vi "test_Checksum U16 - Add Protection.vi"(8 "error in (no error)":errorcluster) -> (0 "error out":errorcluster)   [LabVIEW 2019, in "Protections Unit Tests.lvclass"]
uses:
  Protections Unit Tests.lvclass
  Checksum U16/Checksum U16.lvclass
  <vilib>/addons/_JKI Toolkits/VI Tester/TestCase.llb/TestCase.lvclass
  C:/Program Files (x86)/National Instruments/LabVIEW 2019/vi.lib/addons/_JKI Toolkits/VI Tester/TestCase.llb/TestCase.lvclass
panel:
  out "Checksum U16 out":refnum<class "Checksum U16.lvclass">
  in  "Checksum U16 in":refnum<class "Checksum U16.lvclass">
  out "TestCase out":refnum<class "Protections Unit Tests.lvclass">
  in  "TestCase in":refnum<class "Protections Unit Tests.lvclass">
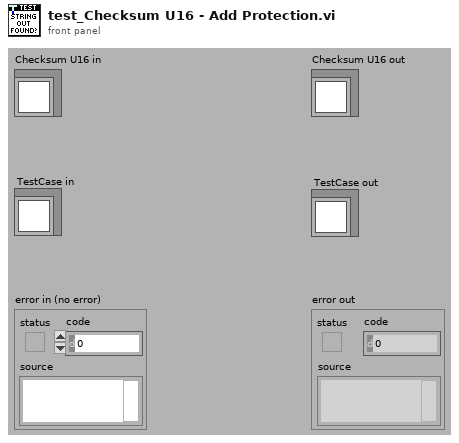
[diagram p1: front panel]
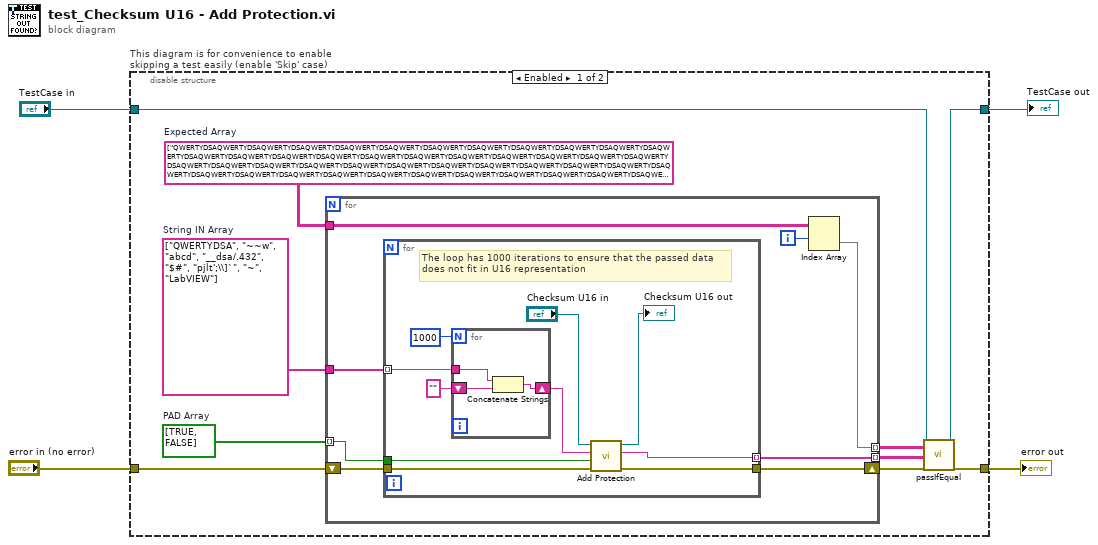
[diagram p0: block diagram]
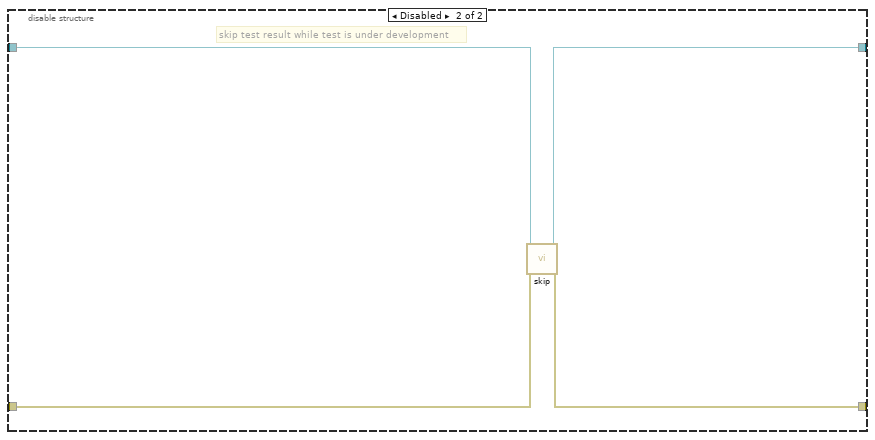
[diagram p2: hidden frame]
diagram:
  n1 = disable-structure "This diagram is for convenience to enable skipping a test easily (enable 'Skip' case)" shown="Enabled" {
    disable-tunnel: "TestCase in" -> [w12 w39]
    disable-tunnel: [w13 w37] -> w1
    disable-tunnel: [w14 w38] -> w3
    disable-tunnel: "error in (no error)" -> [w11 w36]
    frame Enabled {
      w6 = string[][] [["QWERTYDSAQWERTYDSAQWERTYDSAQWERTYDSAQWERTYDSAQWERTYDSAQWERTYDSAQWERTYDSAQWERTYDSAQWERTYDSAQWERTYDSAQWERTYDSAQWERTYDSAQWERTYDSAQWERTYDSAQWERTYDSAQWERTYDSAQWERTYDSAQWERTYDSAQWERTYDSAQWERTYDSAQWERTYDSAQWERTYDSAQWERTYDSAQWERTYDSAQWERTYDSAQWERTYDSAQWERTYDSAQWERTYDSAQWERTYDSAQWERTYDSAQWERTYDSAQWERTYDSAQWERTYDSAQWERTYDSAQWERTYDSAQWERTYDSAQWERTYDSAQWERTYDSAQWERTYDSAQWERTYDSAQWERTYDSAQWERTYDSAQWERTYDSAQWERTYDSAQWERTYDSAQWERTYDSAQWERTYDSAQWERTYDSAQWERTYDSAQWERTYDSAQWERTYDSAQWERTYDSAQWERTYDSAQWERTYDSAQWERTYDSAQWERTYDSAQWERTYDSAQWERTYDSAQWERTYDSAQWERTYDSAQWERTYDSAQWERTYDSAQWERTYDSAQWERTYDSAQWERTYDSAQWERTYDSAQWERTYDSAQWERTYDSAQWERTYDSAQWERTYDSAQWERTYDSAQWERTYDSAQWERTYDSAQWERTYDSAQWERTYDSAQWERTYDSAQWERTYDSAQWERTYDSAQWERTYDSAQWERTYDSAQWERTYDSAQWERTYDSAQWERTYDSAQWERTYDSAQWERTYDSAQWERTYDSAQWERTYDSAQWERTYDSAQWERTYDSAQWERTYDSAQWERTYDSAQWERTYDSAQWERTYDSAQWERTYDSAQWERTYDSAQWERTYDSAQWERTYDSAQWERTYDSAQWERTYDSAQWERTYDSAQWERTYDSAQWERTYDSAQWERTYDSAQWERTYDSAQWERTYDSAQWERTYDSAQWERTYDSAQWERTYDSAQWERTYDSAQWERTYDSAQWERTYDSAQWERTYDSAQWERTYDSAQWERTYDSAQWERTYDSAQWERTYDSAQWERTYDSAQWERTYDSAQWERTYDSAQWERTYDSAQWERTYDSAQWERTYDSAQWERTYDSAQWERTYDSAQWERTYDSAQWERTYDSAQWERTYDSAQWERTYDSAQWERTYDSAQWERTYDSAQWERTYDSAQWERTYDSAQWERTYDSAQWERTYDSAQWERTYDSAQWERTYDSAQWERTYDSAQWERTYDSAQWERTYDSAQWERTYDSAQWERTYDSAQWERTYDSAQWERTYDSAQWERTYDSAQWERTYDSAQWERTYDSAQWERTYDSAQWERTYDSAQWERTYDSAQWERTYDSAQWERTYDSAQWERTYDSAQWERTYDSAQWERTYDSAQWERTYDSAQWERTYDSAQWERTYDSAQWERTYDSAQWERTYDSAQWERTYDSAQWERTYDSAQWERTYDSAQWERTYDSAQWERTYDSAQWERTYDSAQWERTYDSAQWERTYDSAQWERTYDSAQWERTYDSAQWERTYDSAQWERTYDSAQWERTYDSAQWERTYDSAQWERTYDSAQWERTYDSAQWERTYDSAQWERTYDSAQWERTYDSAQWERTYDSAQWERTYDSAQWERTYDSAQWERTYDSAQWERTYDSAQWERTYDSAQWERTYDSAQWERTYDSAQWERTYDSAQWERTYDSAQWERTYDSAQWERTYDSAQWERTYDSAQWERTYDSAQWERTYDSAQWERTYDSAQWERTYDSAQWERTYDSAQWERTYDSAQWERTYDSAQWERTYDSAQWERTYDSAQWERTYDSAQWERTYDSAQWERTYDSAQWERTYDSAQWERTYDSAQWERTYDSAQWERTYDSAQWERTYDSAQWERTYDSAQWERTYDSAQWERTYDSAQWERTYDSAQWERTYDSAQWERTYDSAQWERTYDSAQWERTYDSAQWERTYDSAQWERTYDSAQWERTYDSAQWERTYDSAQWERTYDSAQWERTYDSAQWERTYDSAQWERTYDSAQWERTYDSAQWERTYDSAQWERTYDSAQWERTYDSAQWERTYDSAQWERTYDSAQWERTYDSAQWERTYDSAQWERTYDSAQWERTYDSAQWERTYDSAQWERTYDSAQWERTYDSAQWERTYDSAQWERTYDSAQWERTYDSAQWERTYDSAQWERTYDSAQWERTYDSAQWERTYDSAQWERTYDSAQWERTYDSAQWERTYDSAQWERTYDSAQWERTYDSAQWERTYDSAQWERTYDSAQWERTYDSAQWERTYDSAQWERTYDSAQWERTYDSAQWERTYDSAQWERTYDSAQWERTYDSAQWERTYDSAQWERTYDSAQWERTYDSAQWERTYDSAQWERTYDSAQWERTYDSAQWERTYDSAQWERTYDSAQWERTYDSAQWERTYDSAQWERTYDSAQWERTYDSAQWERTYDSAQWERTYDSAQWERTYDSAQWERTYDSAQWERTYDSAQWERTYDSAQWERTYDSAQWERTYDSAQWERTYDSAQWERTYDSAQWERTYDSAQWERTYDSAQWERTYDSAQWERTYDSAQWERTYDSAQWERTYDSAQWERTYDSAQWERTYDSAQWERTYDSAQWERTYDSAQWERTYDSAQWERTYDSAQWERTYDSAQWERTYDSAQWERTYDSAQWERTYDSAQWERTYDSAQWERTYDSAQWERTYDSAQWERTYDSAQWERTYDSAQWERTYDSAQWERTYDSAQWERTYDSAQWERTYDSAQWERTYDSAQWERTYDSAQWERTYDSAQWERTYDSAQWERTYDSAQWERTYDSAQWERTYDSAQWERTYDSAQWERTYDSAQWERTYDSAQWERTYDSAQWERTYDSAQWERTYDSAQWERTYDSAQWERTYDSAQWERTYDSAQWERTYDSAQWERTYDSAQWERTYDSAQWERTYDSAQWERTYDSAQWERTYDSAQWERTYDSAQWERTYDSAQWERTYDSAQWERTYDSAQWERTYDSAQWERTYDSAQWERTYDSAQWERTYDSAQWERTYDSAQWERTYDSAQWERTYDSAQWERTYDSAQWERTYDSAQWERTYDSAQWERTYDSAQWERTYDSAQWERTYDSAQWERTYDSAQWERTYDSAQWERTYDSAQWERTYDSAQWERTYDSAQWERTYDSAQWERTYDSAQWERTYDSAQWERTYDSAQWERTYDSAQWERTYDSAQWERTYDSAQWERTYDSAQWERTYDSAQWERTYDSAQWERTYDSAQWERTYDSAQWERTYDSAQWERTYDSAQWERTYDSAQWERTYDSAQWERTYDSAQWERTYDSAQWERTYDSAQWERTYDSAQWERTYDSAQWERTYDSAQWERTYDSAQWERTYDSAQWERTYDSAQWERTYDSAQWERTYDSAQWERTYDSAQWERTYDSAQWERTYDSAQWERTYDSAQWERTYDSAQWERTYDSAQWERTYDSAQWERTYDSAQWERTYDSAQWERTYDSAQWERTYDSAQWERTYDSAQWERTYDSAQWERTYDSAQWERTYDSAQWERTYDSAQWERTYDSAQWERTYDSAQWERTYDSAQWERTYDSAQWERTYDSAQWERTYDSAQWERTYDSAQWERTYDSAQWERTYDSAQWERTYDSAQWERTYDSAQWERTYDSAQWERTYDSAQWERTYDSAQWERTYDSAQWERTYDSAQWERTYDSAQWERTYDSAQWERTYDSAQWERTYDSAQWERTYDSAQWERTYDSAQWERTYDSAQWERTYDSAQWERTYDSAQWERTYDSAQWERTYDSAQWERTYDSAQWERTYDSAQWERTYDSAQWERTYDSAQWERTYDSAQWERTYDSAQWERTYDSAQWERTYDSAQWERTYDSAQWERTYDSAQWERTYDSAQWERTYDSAQWERTYDSAQWERTYDSAQWERTYDSAQWERTYDSAQWERTYDSAQWERTYDSAQWERTYDSAQWERTYDSAQWERTYDSAQWERTYDSAQWERTYDSAQWERTYDSAQWERTYDSAQWERTYDSAQWERTYDSAQWERTYDSAQWERTYDSAQWERTYDSAQWERTYDSAQWERTYDSAQWERTYDSAQWERTYDSAQWERTYDSAQWERTYDSAQWERTYDSAQWERTYDSAQWERTYDSAQWERTYDSAQWERTYDSAQWERTYDSAQWERTYDSAQWERTYDSAQWERTYDSAQWERTYDSAQWERTYDSAQWERTYDSAQWERTYDSAQWERTYDSAQWERTYDSAQWERTYDSAQWERTYDSAQWERTYDSAQWERTYDSAQWERTYDSAQWERTYDSAQWERTYDSAQWERTYDSAQWERTYDSAQWERTYDSAQWERTYDSAQWERTYDSAQWERTYDSAQWERTYDSAQWERTYDSAQWERTYDSAQWERTYDSAQWERTYDSAQWERTYDSAQWERTYDSAQWERTYDSAQWERTYDSAQWERTYDSAQWERTYDSAQWERTYDSAQWERTYDSAQWERTYDSAQWERTYDSAQWERTYDSAQWERTYDSAQWERTYDSAQWERTYDSAQWERTYDSAQWERTYDSAQWERTYDSAQWERTYDSAQWERTYDSAQWERTYDSAQWERTYDSAQWERTYDSAQWERTYDSAQWERTYDSAQWERTYDSAQWERTYDSAQWERTYDSAQWERTYDSAQWERTYDSAQWERTYDSAQWERTYDSAQWERTYDSAQWERTYDSAQWERTYDSAQWERTYDSAQWERTYDSAQWERTYDSAQWERTYDSAQWERTYDSAQWERTYDSAQWERTYDSAQWERTYDSAQWERTYDSAQWERTYDSAQWERTYDSAQWERTYDSAQWERTYDSAQWERTYDSAQWERTYDSAQWERTYDSAQWERTYDSAQWERTYDSAQWERTYDSAQWERTYDSAQWERTYDSAQWERTYDSAQWERTYDSAQWERTYDSAQWERTYDSAQWERTYDSAQWERTYDSAQWERTYDSAQWERTYDSAQWERTYDSAQWERTYDSAQWERTYDSAQWERTYDSAQWERTYDSAQWERTYDSAQWERTYDSAQWERTYDSAQWERTYDSAQWERTYDSAQWERTYDSAQWERTYDSAQWERTYDSAQWERTYDSAQWERTYDSAQWERTYDSAQWERTYDSAQWERTYDSAQWERTYDSAQWERTYDSAQWERTYDSAQWERTYDSAQWERTYDSAQWERTYDSAQWERTYDSAQWERTYDSAQWERTYDSAQWERTYDSAQWERTYDSAQWERTYDSAQWERTYDSAQWERTYDSAQWERTYDSAQWERTYDSAQWERTYDSAQWERTYDSAQWERTYDSAQWERTYDSAQWERTYDSAQWERTYDSAQWERTYDSAQWERTYDSAQWERTYDSAQWERTYDSAQWERTYDSAQWERTYDSAQWERTYDSAQWERTYDSAQWERTYDSAQWERTYDSAQWERTYDSAQWERTYDSAQWERTYDSAQWERTYDSAQWERTYDSAQWERTYDSAQWERTYDSAQWERTYDSAQWERTYDSAQWERTYDSAQWERTYDSAQWERTYDSAQWERTYDSAQWERTYDSAQWERTYDSAQWERTYDSAQWERTYDSAQWERTYDSAQWERTYDSAQWERTYDSAQWERTYDSAQWERTYDSAQWERTYDSAQWERTYDSAQWERTYDSAQWERTYDSAQWERTYDSAQWERTYDSAQWERTYDSAQWERTYDSAQWERTYDSAQWERTYDSAQWERTYDSAQWERTYDSAQWERTYDSAQWERTYDSAQWERTYDSAQWERTYDSAQWERTYDSAQWERTYDSAQWERTYDSAQWERTYDSAQWERTYDSAQWERTYDSAQWERTYDSAQWERTYDSAQWERTYDSAQWERTYDSAQWERTYDSAQWERTYDSAQWERTYDSAQWERTYDSAQWERTYDSAQWERTYDSAQWERTYDSAQWERTYDSAQWERTYDSAQWERTYDSAQWERTYDSAQWERTYDSAQWERTYDSAQWERTYDSAQWERTYDSAQWERTYDSAQWERTYDSAQWERTYDSAQWERTYDSAQWERTYDSAQWERTYDSAQWERTYDSAQWERTYDSAQWERTYDSAQWERTYDSAQWERTYDSAQWERTYDSAQWERTYDSAQWERTYDSAQWERTYDSAQWERTYDSAQWERTYDSAQWERTYDSAQWERTYDSAQWERTYDSAQWERTYDSAQWERTYDSAQWERTYDSAQWERTYDSAQWERTYDSAQWERTYDSAQWERTYDSAQWERTYDSAQWERTYDSAQWERTYDSAQWERTYDSAQWERTYDSAQWERTYDSAQWERTYDSAQWERTYDSAQWERTYDSAQWERTYDSAQWERTYDSAQWERTYDSAQWERTYDSAQWERTYDSAQWERTYDSAQWERTYDSAQWERTYDSAQWERTYDSAQWERTYDSAQWERTYDSAQWERTYDSAQWERTYDSAQWERTYDSAQWERTYDSAQWERTYDSAQWERTYDSAQWERTYDSAQWERTYDSAQWERTYDSAQWERTYDSAQWERTYDSAQWERTYDSAQWERTYDSAQWERTYDSAQWERTYDSAQWERTYDSAQWERTYDSAQWERTYDSAQWERTYDSAQWERTYDSAQWERTYDSAQWERTYDSAQWERTYDSAQWERTYDSAQWERTYDSAQWERTYDSAQWERTYDSAQWERTYDSAQWERTYDSAQWERTYDSAQWERTYDSAQWERTYDSAQWERTYDSAQWERTYDSAQWERTYDSAQWERTYDSAQWERTYDSAQWERTYDSAQWERTYDSAQWERTYDSAQWERTYDSAQWERTYDSAQWERTYDSAQWERTYDSAQWERTYDSAQWERTYDSAQWERTYDSAQWERTYDSAQWERTYDSAQWERTYDSAQWERTYDSAQWERTYDSAQWERTYDSAQWERTYDSAQWERTYDSAQWERTYDSAQWERTYDSAQWERTYDSAQWERTYDSAQWERTYDSAQWERTYDSAQWERTYDSAQWERTYDSAQWERTYDSAQWERTYDSAQWERTYDSAQWERTYDSAQWERTYDSAQWERTYDSAQWERTYDSAQWERTYDSAQWERTYDSAQWERTYDSAQWERTYDSAQWERTYDSAQWERTYDSAQWERTYDSAQWERTYDSAQWERTYDSAQWERTYDSAQWERTYDSAQWERTYDSAQWERTYDSAQWERTYDSAQWERTYDSAQWERTYDSAQWERTYDSAQWERTYDSAQWERTYDSAQWERTYDSAQWERTYDSAQWERTYDSAQWERTYDSAQWERTYDSAQWERTYDSAQWERTYDSAQWERTYDSAQWERTYDSAQWERTYDSAQWERTYDSAQWERTYDSAQWERTYDSAQWERTYDSAQWERTYDSAQWERTYDSAQWERTYDSAQWERTYDSAQWERTYDSAQWERTYDSAQWERTYDSAQWERTYDSAQWERTYDSAQWERTYDSAQWERTYDSAQWERTYDSAQWERTYDSAQWERTYDSAQWERTYDSAQWERTYDSAQWERTYDSAQWERTYDSAQWERTYDSAQWERTYDSAQWERTYDSAQWERTYDSAQWERTYDSAQWERTYDSAQWERTYDSAQWERTYDSAQWERTYDSAQWERTYDSAQWERTYDSAQWERTYDSAQWERTYDSAQWERTYDSAQWERTYDSAQWERTYDSAQWERTYDSAQWERTYDSAQWERTYDSAQWERTYDSAQWERTYDSAQWERTYDSAQWERTYDSAQWERTYDSAQWERTYDSAQWERTYDSAQWERTYDSAQWERTYDSAQWERTYDSAQWERTYDSAQWERTYDSAQWERTYDSAQWERTYDSAQWERTYDSAQWERTYDSAQWERTYDSAQWERTYDSAQWERTYDSAQWERTYDSAQWERTYDSAQWERTYDSAQWERTYDSAQWERTYDSAQWERTYDSAQWERTYDSAQWERTYDSAQWERTYDSAQWERTYDSAQWERTYDSAQWERTYDSAQWERTYDSAQWERTYDSAQWERTYDSAQWERTYDSAQWERTYDSAQWERTYDSAQWERTYDSAQWERTYDSAQWERTYDSAQWERTYDSAQWERTYDSAQWERTYDSAQWERTYDSAQWERTYDSAQWERTYDSAQWERTYDSAQWERTYDSAQWERTYDSAQWERTYDSAQWERTYDSAQWERTYDSAQWERTYDSAQWERTYDSAQWERTYDSAQWERTYDSAQWERTYDSAQWERTYDSAQWERTYDSAQWERTYDSAQWERTYDSAQWERTYDSAQWERTYDSAQWERTYDSAQWERTYDSAQWERTYDSAQWERTYDSAQWERTYDSAQWERTYDSAQWERTYDSAQWERTYDSAQWERTYDSAQWERTYDSAQWERTYDSAQWERTYDSAQWERTYDSAQWERTYDSAQWERTYDSAQWERTYDSAQWERTYDSAQWERTYDSAQWERTYDSAQWERTYDSAQWERTYDSAQWERTYDSAQWERTYDSAQWERTYDSAQWERTYDSAQWERTYDSAQWERTYDSAQWERTYDSAQWERTYDSAQWERTYDSAQWERTYDSAQWERTYDSAQWERTYDSAQWERTYDSAQWERTYDSAQWERTYDSAQWERTYDSAQWERTYDSAQWERTYDSAQWERTYDSAQWERTYDSAQWERTYDSAQWERTYDSAQWERTYDSAQWERTYDSAQWERTYDSAQWERTYDSAQWERTYDSAQWERTYDSAQWERTYDSAQWERTYDSAQWERTYDSAQWERTYDSAQWERTYDSAQWERTYDSAQWERTYDSAQWERTYDSAQWERTYDSAQWERTYDSAQWERTYDSAQWERTYDSAQWERTYDSAQWERTYDSAQWERTYDSAQWERTYDSAQWERTYDSAQWERTYDSAQWERTYDSAQWERTYDSAQWERTYDSAQWERTYDSAQWERTYDSAQWERTYDSAQWERTYDSAQWERTYDSAQWERTYDSAQWERTYDSAQWERTYDSAQWERTYDSAQWERTYDSAQWERTYDSAQWERTYDSAQWERTYDSAQWERTYDSAQWERTYD͠", "~~w~~w~~w~~w~~w~~w~~w~~w~~w~~w~~w~~w~~w~~w~~w~~w~~w~~w~~w~~w~~w~~w~~w~~w~~w~~w~~w~~w~~w~~w~~w~~w~~w~~w~~w~~w~~w~~w~~w~~w~~w~~w~~w~~w~~w~~w~~w~~w~~w~~w~~w~~w~~w~~w~~w~~w~~w~~w~~w~~w~~w~~w~~w~~w~~w~~w~~w~~w~~w~~w~~w~~w~~w~~w~~w~~w~~w~~w~~w~~w~~w~~w~~w~~w~~w~~w~~w~~w~~w~~w~~w~~w~~w~~w~~w~~w~~w~~w~~w~~w~~w~~w~~w~~w~~w~~w~~w~~w~~w~~w~~w~~w~~w~~w~~w~~w~~w~~w~~w~~w~~w~~w~~w~~w~~w~~w~~w~~w~~w~~w~~w~~w~~w~~w~~w~~w~~w~~w~~w~~w~~w~~w~~w~~w~~w~~w~~w~~w~~w~~w~~w~~w~~w~~w~~w~~w~~w~~w~~w~~w~~w~~w~~w~~w~~w~~w~~w~~w~~w~~w~~w~~w~~w~~w~~w~~w~~w~~w~~w~~w~~w~~w~~w~~w~~w~~w~~w~~w~~w~~w~~w~~w~~w~~w~~w~~w~~w~~w~~w~~w~~w~~w~~w~~w~~w~~w~~w~~w~~w~~w~~w~~w~~w~~w~~w~~w~~w~~w~~w~~w~~w~~w~~w~~w~~w~~w~~w~~w~~w~~w~~w~~w~~w~~w~~w~~w~~w~~w~~w~~w~~w~~w~~w~~w~~w~~w~~w~~w~~w~~w~~w~~w~~w~~w~~w~~w~~w~~w~~w~~w~~w~~w~~w~~w~~w~~w~~w~~w~~w~~w~~w~~w~~w~~w~~w~~w~~w~~w~~w~~w~~w~~w~~w~~w~~w~~w~~w~~w~~w~~w~~w~~w~~w~~w~~w~~w~~w~~w~~w~~w~~w~~w~~w~~w~~w~~w~~w~~w~~w~~w~~w~~w~~w~~w~~w~~w~~w~~w~~w~~w~~w~~w~~w~~w~~w~~w~~w~~w~~w~~w~~w~~w~~w~~w~~w~~w~~w~~w~~w~~w~~w~~w~~w~~w~~w~~w~~w~~w~~w~~w~~w~~w~~w~~w~~w~~w~~w~~w~~w~~w~~w~~w~~w~~w~~w~~w~~w~~w~~w~~w~~w~~w~~w~~w~~w~~w~~w~~w~~w~~w~~w~~w~~w~~w~~w~~w~~w~~w~~w~~w~~w~~w~~w~~w~~w~~w~~w~~w~~w~~w~~w~~w~~w~~w~~w~~w~~w~~w~~w~~w~~w~~w~~w~~w~~w~~w~~w~~w~~w~~w~~w~~w~~w~~w~~w~~w~~w~~w~~w~~w~~w~~w~~w~~w~~w~~w~~w~~w~~w~~w~~w~~w~~w~~w~~w~~w~~w~~w~~w~~w~~w~~w~~w~~w~~w~~w~~w~~w~~w~~w~~w~~w~~w~~w~~w~~w~~w~~w~~w~~w~~w~~w~~w~~w~~w~~w~~w~~w~~w~~w~~w~~w~~w~~w~~w~~w~~w~~w~~w~~w~~w~~w~~w~~w~~w~~w~~w~~w~~w~~w~~w~~w~~w~~w~~w~~w~~w~~w~~w~~w~~w~~w~~w~~w~~w~~w~~w~~w~~w~~w~~w~~w~~w~~w~~w~~w~~w~~w~~w~~w~~w~~w~~w~~w~~w~~w~~w~~w~~w~~w~~w~~w~~w~~w~~w~~w~~w~~w~~w~~w~~w~~w~~w~~w~~w~~w~~w~~w~~w~~w~~w~~w~~w~~w~~w~~w~~w~~w~~w~~w~~w~~w~~w~~w~~w~~w~~w~~w~~w~~w~~w~~w~~w~~w~~w~~w~~w~~w~~w~~w~~w~~w~~w~~w~~w~~w~~w~~w~~w~~w~~w~~w~~w~~w~~w~~w~~w~~w~~w~~w~~w~~w~~w~~w~~w~~w~~w~~w~~w~~w~~w~~w~~w~~w~~w~~w~~w~~w~~w~~w~~w~~w~~w~~w~~w~~w~~w~~w~~w~~w~~w~~w~~w~~w~~w~~w~~w~~w~~w~~w~~w~~w~~w~~w~~w~~w~~w~~w~~w~~w~~w~~w~~w~~w~~w~~w~~w~~w~~w~~w~~w~~w~~w~~w~~w~~w~~w~~w~~w~~w~~w~~w~~w~~w~~w~~w~~w~~w~~w~~w~~w~~w~~w~~w~~w~~w~~w~~w~~w~~w~~w~~w~~w~~w~~w~~w~~w~~w~~w~~w~~w~~w~~w~~w~~w~~w~~w~~w~~w~~w~~w~~w~~w~~w~~w~~w~~w~~w~~w~~w~~w~~w~~w~~w~~w~~w~~w~~w~~w~~w~~w~~w~~w~~w~~w~~w~~w~~w~~w~~w~~w~~w~~w~~w~~w~~w~~w~~w~~w~~w~~w~~w~~w~~w~~w~~w~~w~~w~~w~~w~~w~~w~~w~~w~~w~~w~~w~~w~~w~~w~~w~~w~~w~~w~~w~~w~~w~~w~~w~~w~~w~~w~~w~~w~~w~~w~~w~~w~~w~~w~~w~~w~~w~~w~~w~~w~~w~~w~~w~~w~~w~~w~~w~~w~~w~~w~~w~~w~~w~~w~~w~~w~~w~~w~~w~~w~~w~~w~~w~~w~~w~~w~~w~~w~~w~~w~~w~~w~~w~~w~~w~~w~~w~~w~~w~~w~~w~~w~~w~~w~~w~~w~~w~~w~~w~~w~~w~~w~~w~~w~~w~~w~~w~~w~~w~~w~~w~~w~~w~~w~~w~~w~~w~~w~~w~~w~~w~~w~~w~~w~~w~~w~~w~~w~~w~~w~~w~~w~~w~~w~~w~~w~~w~~w~~w~~w~~w~~w~~w~~w~~w~~w~~w~~w~~w~~w~~w~~w~~w~~w~~w~~w~~w~~w~~w~~w~~w~~w~~w~~w~~w~~w~~w~~w~~w~~w~~w~~w~~w~~w~~w~~w~~w~~w~~w~~w~~w~~w~~w~~w~~w~~w~~w~~w~~w~~w~~w~~w~~w~~w~~w~~w~~w~~w~~w~~w~~w~~w~~w~~w~~w~~w~~w~~w~~w~~w~~w~~w~~w~~w~~w~~w~~w~~w~~w~~w~~w~~w~~w~~w~~w~~w~~w~~w~~w~~w~~w~~w~~w~~w~~w~~w~~w~~w~~w~~w~~w~~w~~w~©8", "abcdabcdabcdabcdabcdabcdabcdabcdabcdabcdabcdabcdabcdabcdabcdabcdabcdabcdabcdabcdabcdabcdabcdabcdabcdabcdabcdabcdabcdabcdabcdabcdabcdabcdabcdabcdabcdabcdabcdabcdabcdabcdabcdabcdabcdabcdabcdabcdabcdabcdabcdabcdabcdabcdabcdabcdabcdabcdabcdabcdabcdabcdabcdabcdabcdabcdabcdabcdabcdabcdabcdabcdabcdabcdabcdabcdabcdabcdabcdabcdabcdabcdabcdabcdabcdabcdabcdabcdabcdabcdabcdabcdabcdabcdabcdabcdabcdabcdabcdabcdabcdabcdabcdabcdabcdabcdabcdabcdabcdabcdabcdabcdabcdabcdabcdabcdabcdabcdabcdabcdabcdabcdabcdabcdabcdabcdabcdabcdabcdabcdabcdabcdabcdabcdabcdabcdabcdabcdabcdabcdabcdabcdabcdabcdabcdabcdabcdabcdabcdabcdabcdabcdabcdabcdabcdabcdabcdabcdabcdabcdabcdabcdabcdabcdabcdabcdabcdabcdabcdabcdabcdabcdabcdabcdabcdabcdabcdabcdabcdabcdabcdabcdabcdabcdabcdabcdabcdabcdabcdabcdabcdabcdabcdabcdabcdabcdabcdabcdabcdabcdabcdabcdabcdabcdabcdabcdabcdabcdabcdabcdabcdabcdabcdabcdabcdabcdabcdabcdabcdabcdabcdabcdabcdabcdabcdabcdabcdabcdabcdabcdabcdabcdabcdabcdabcdabcdabcdabcdabcdabcdabcdabcdabcdabcdabcdabcdabcdabcdabcdabcdabcdabcdabcdabcdabcdabcdabcdabcdabcdabcdabcdabcdabcdabcdabcdabcdabcdabcdabcdabcdabcdabcdabcdabcdabcdabcdabcdabcdabcdabcdabcdabcdabcdabcdabcdabcdabcdabcdabcdabcdabcdabcdabcdabcdabcdabcdabcdabcdabcdabcdabcdabcdabcdabcdabcdabcdabcdabcdabcdabcdabcdabcdabcdabcdabcdabcdabcdabcdabcdabcdabcdabcdabcdabcdabcdabcdabcdabcdabcdabcdabcdabcdabcdabcdabcdabcdabcdabcdabcdabcdabcdabcdabcdabcdabcdabcdabcdabcdabcdabcdabcdabcdabcdabcdabcdabcdabcdabcdabcdabcdabcdabcdabcdabcdabcdabcdabcdabcdabcdabcdabcdabcdabcdabcdabcdabcdabcdabcdabcdabcdabcdabcdabcdabcdabcdabcdabcdabcdabcdabcdabcdabcdabcdabcdabcdabcdabcdabcdabcdabcdabcdabcdabcdabcdabcdabcdabcdabcdabcdabcdabcdabcdabcdabcdabcdabcdabcdabcdabcdabcdabcdabcdabcdabcdabcdabcdabcdabcdabcdabcdabcdabcdabcdabcdabcdabcdabcdabcdabcdabcdabcdabcdabcdabcdabcdabcdabcdabcdabcdabcdabcdabcdabcdabcdabcdabcdabcdabcdabcdabcdabcdabcdabcdabcdabcdabcdabcdabcdabcdabcdabcdabcdabcdabcdabcdabcdabcdabcdabcdabcdabcdabcdabcdabcdabcdabcdabcdabcdabcdabcdabcdabcdabcdabcdabcdabcdabcdabcdabcdabcdabcdabcdabcdabcdabcdabcdabcdabcdabcdabcdabcdabcdabcdabcdabcdabcdabcdabcdabcdabcdabcdabcdabcdabcdabcdabcdabcdabcdabcdabcdabcdabcdabcdabcdabcdabcdabcdabcdabcdabcdabcdabcdabcdabcdabcdabcdabcdabcdabcdabcdabcdabcdabcdabcdabcdabcdabcdabcdabcdabcdabcdabcdabcdabcdabcdabcdabcdabcdabcdabcdabcdabcdabcdabcdabcdabcdabcdabcdabcdabcdabcdabcdabcdabcdabcdabcdabcdabcdabcdabcdabcdabcdabcdabcdabcdabcdabcdabcdabcdabcdabcdabcdabcdabcdabcdabcdabcdabcdabcdabcdabcdabcdabcdabcdabcdabcdabcdabcdabcdabcdabcdabcdabcdabcdabcdabcdabcdabcdabcdabcdabcdabcdabcdabcdabcdabcdabcdabcdabcdabcdabcdabcdabcdabcdabcdabcdabcdabcdabcdabcdabcdabcdabcdabcdabcdabcdabcdabcdabcdabcdabcdabcdabcdabcdabcdabcdabcdabcdabcdabcdabcdabcdabcdabcdabcdabcdabcdabcdabcdabcdabcdabcdabcdabcdabcdabcdabcdabcdabcdabcdabcdabcdabcdabcdabcdabcdabcdabcdabcdabcdabcdabcdabcdabcdabcdabcdabcdabcdabcdabcdabcdabcdabcdabcdabcdabcdabcdabcdabcdabcdabcdabcdabcdabcdabcdabcdabcdabcdabcdabcdabcdabcdabcdabcdabcdabcdabcdabcdabcdabcdabcdabcdabcdabcdabcdabcdabcdabcdabcdabcdabcdabcdabcdabcdabcdabcdabcdabcdabcdabcdabcdabcdabcdabcdabcdabcdabcdabcdabcdabcdabcdabcdabcdabcdabcdabcdabcdabcdabcdabcdabcdabcdabcdabcdabcdabcdabcdabcdabcdabcdabcdabcdabcdabcdabcdabcdabcdabcdabcdabcdabcdabcdabcdabcdabcdabcdabcdabcdabcdabcdabcdabcdabcdabcdabcdabcdabcdabcdabcdabcdabcdabcdabcdabcdabcdabcdabcdabcdabcdabcdabcdabcdabcdabcdabcdabcdabcdabcdabcdabcdabcdabcdabcdabcdabcdabcdabcdabcdabcdabcdabcdabcdabcdabcdabcdabcdabcdabcdabcdabcdabcdabcdabcdabcdabcdabcdabcdabcdabcdabcdabcdabcdabcdabcdabcdabcdabcdabcdabcdabcdabcdabcdabcdabcdabcdabcdabcdabcdabcdabcdabcdabcdabcdabcdabcdabcdabcdabcdabcdabcdabcdabcdabcdabcdabcdabcdabcdabcdabcdabcdabcdabcdabcdabcdabcdabcdabcdabcdabcdabcdabcdabcdabcdabcdabcdabcdabcdabcdabcdabcdabcdabcdabcdabcdabcdabcdabcdabcdabcdabcdabcdabcdabcdabcdabcdabcdabcdabcdabcdabcdabcdabcdabcdabcdabcdabcdabcdabcdabcdabcdabcdabcdabcdabcdabcdabcdabcdabcdabcdabcdabcdabcdabcdabcdabcdabcdabcdabcdabcdabcdabcdabcdabcdabcdabcdabcdabcdabcdabcdabcdabcdabcdabcdabcdabcdabcdabcdabcdabcdab\u0003\u0010", "__dsa/.432__dsa/.432__dsa/.432__dsa/.432__dsa/.432__dsa/.432__dsa/.432__dsa/.432__dsa/.432__dsa/.432__dsa/.432__dsa/.432__dsa/.432__dsa/.432__dsa/.432__dsa/.432__dsa/.432__dsa/.432__dsa/.432__dsa/.432__dsa/.432__dsa/.432__dsa/.432__dsa/.432__dsa/.432__dsa/.432__dsa/.432__dsa/.432__dsa/.432__dsa/.432__dsa/.432__dsa/.432__dsa/.432__dsa/.432__dsa/.432__dsa/.432__dsa/.432__dsa/.432__dsa/.432__dsa/.432__dsa/.432__dsa/.432__dsa/.432__dsa/.432__dsa/.432__dsa/.432__dsa/.432__dsa/.432__dsa/.432__dsa/.432__dsa/.432__dsa/.432__dsa/.432__dsa/.432__dsa/.432__dsa/.432__dsa/.432__dsa/.432__dsa/.432__dsa/.432__dsa/.432__dsa/.432__dsa/.432__dsa/.432__dsa/.432__dsa/.432__dsa/.432__dsa/.432__dsa/.432__dsa/.432__dsa/.432__dsa/.432__dsa/.432__dsa/.432__dsa/.432__dsa/.432__dsa/.432__dsa/.432__dsa/.432__dsa/.432__dsa/.432__dsa/.432__dsa/.432__dsa/.432__dsa/.432__dsa/.432__dsa/.432__dsa/.432__dsa/.432__dsa/.432__dsa/.432__dsa/.432__dsa/.432__dsa/.432__dsa/.432__dsa/.432__dsa/.432__dsa/.432__dsa/.432__dsa/.432__dsa/.432__dsa/.432__dsa/.432__dsa/.432__dsa/.432__dsa/.432__dsa/.432__dsa/.432__dsa/.432__dsa/.432__dsa/.432__dsa/.432__dsa/.432__dsa/.432__dsa/.432__dsa/.432__dsa/.432__dsa/.432__dsa/.432__dsa/.432__dsa/.432__dsa/.432__dsa/.432__dsa/.432__dsa/.432__dsa/.432__dsa/.432__dsa/.432__dsa/.432__dsa/.432__dsa/.432__dsa/.432__dsa/.432__dsa/.432__dsa/.432__dsa/.432__dsa/.432__dsa/.432__dsa/.432__dsa/.432__dsa/.432__dsa/.432__dsa/.432__dsa/.432__dsa/.432__dsa/.432__dsa/.432__dsa/.432__dsa/.432__dsa/.432__dsa/.432__dsa/.432__dsa/.432__dsa/.432__dsa/.432__dsa/.432__dsa/.432__dsa/.432__dsa/.432__dsa/.432__dsa/.432__dsa/.432__dsa/.432__dsa/.432__dsa/.432__dsa/.432__dsa/.432__dsa/.432__dsa/.432__dsa/.432__dsa/.432__dsa/.432__dsa/.432__dsa/.432__dsa/.432__dsa/.432__dsa/.432__dsa/.432__dsa/.432__dsa/.432__dsa/.432__dsa/.432__dsa/.432__dsa/.432__dsa/.432__dsa/.432__dsa/.432__dsa/.432__dsa/.432__dsa/.432__dsa/.432__dsa/.432__dsa/.432__dsa/.432__dsa/.432__dsa/.432__dsa/.432__dsa/.432__dsa/.432__dsa/.432__dsa/.432__dsa/.432__dsa/.432__dsa/.432__dsa/.432__dsa/.432__dsa/.432__dsa/.432__dsa/.432__dsa/.432__dsa/.432__dsa/.432__dsa/.432__dsa/.432__dsa/.432__dsa/.432__dsa/.432__dsa/.432__dsa/.432__dsa/.432__dsa/.432__dsa/.432__dsa/.432__dsa/.432__dsa/.432__dsa/.432__dsa/.432__dsa/.432__dsa/.432__dsa/.432__dsa/.432__dsa/.432__dsa/.432__dsa/.432__dsa/.432__dsa/.432__dsa/.432__dsa/.432__dsa/.432__dsa/.432__dsa/.432__dsa/.432__dsa/.432__dsa/.432__dsa/.432__dsa/.432__dsa/.432__dsa/.432__dsa/.432__dsa/.432__dsa/.432__dsa/.432__dsa/.432__dsa/.432__dsa/.432__dsa/.432__dsa/.432__dsa/.432__dsa/.432__dsa/.432__dsa/.432__dsa/.432__dsa/.432__dsa/.432__dsa/.432__dsa/.432__dsa/.432__dsa/.432__dsa/.432__dsa/.432__dsa/.432__dsa/.432__dsa/.432__dsa/.432__dsa/.432__dsa/.432__dsa/.432__dsa/.432__dsa/.432__dsa/.432__dsa/.432__dsa/.432__dsa/.432__dsa/.432__dsa/.432__dsa/.432__dsa/.432__dsa/.432__dsa/.432__dsa/.432__dsa/.432__dsa/.432__dsa/.432__dsa/.432__dsa/.432__dsa/.432__dsa/.432__dsa/.432__dsa/.432__dsa/.432__dsa/.432__dsa/.432__dsa/.432__dsa/.432__dsa/.432__dsa/.432__dsa/.432__dsa/.432__dsa/.432__dsa/.432__dsa/.432__dsa/.432__dsa/.432__dsa/.432__dsa/.432__dsa/.432__dsa/.432__dsa/.432__dsa/.432__dsa/.432__dsa/.432__dsa/.432__dsa/.432__dsa/.432__dsa/.432__dsa/.432__dsa/.432__dsa/.432__dsa/.432__dsa/.432__dsa/.432__dsa/.432__dsa/.432__dsa/.432__dsa/.432__dsa/.432__dsa/.432__dsa/.432__dsa/.432__dsa/.432__dsa/.432__dsa/.432__dsa/.432__dsa/.432__dsa/.432__dsa/.432__dsa/.432__dsa/.432__dsa/.432__dsa/.432__dsa/.432__dsa/.432__dsa/.432__dsa/.432__dsa/.432__dsa/.432__dsa/.432__dsa/.432__dsa/.432__dsa/.432__dsa/.432__dsa/.432__dsa/.432__dsa/.432__dsa/.432__dsa/.432__dsa/.432__dsa/.432__dsa/.432__dsa/.432__dsa/.432__dsa/.432__dsa/.432__dsa/.432__dsa/.432__dsa/.432__dsa/.432__dsa/.432__dsa/.432__dsa/.432__dsa/.432__dsa/.432__dsa/.432__dsa/.432__dsa/.432__dsa/.432__dsa/.432__dsa/.432__dsa/.432__dsa/.432__dsa/.432__dsa/.432__dsa/.432__dsa/.432__dsa/.432__dsa/.432__dsa/.432__dsa/.432__dsa/.432__dsa/.432__dsa/.432__dsa/.432__dsa/.432__dsa/.432__dsa/.432__dsa/.432__dsa/.432__dsa/.432__dsa/.432__dsa/.432__dsa/.432__dsa/.432__dsa/.432__dsa/.432__dsa/.432__dsa/.432__dsa/.432__dsa/.432__dsa/.432__dsa/.432__dsa/.432__dsa/.432__dsa/.432__dsa/.432__dsa/.432__dsa/.432__dsa/.432__dsa/.432__dsa/.432__dsa/.432__dsa/.432__dsa/.432__dsa/.432__dsa/.432__dsa/.432__dsa/.432__dsa/.432__dsa/.432__dsa/.432__dsa/.432__dsa/.432__dsa/.432__dsa/.432__dsa/.432__dsa/.432__dsa/.432__dsa/.432__dsa/.432__dsa/.432__dsa/.432__dsa/.432__dsa/.432__dsa/.432__dsa/.432__dsa/.432__dsa/.432__dsa/.432__dsa/.432__dsa/.432__dsa/.432__dsa/.432__dsa/.432__dsa/.432__dsa/.432__dsa/.432__dsa/.432__dsa/.432__dsa/.432__dsa/.432__dsa/.432__dsa/.432__dsa/.432__dsa/.432__dsa/.432__dsa/.432__dsa/.432__dsa/.432__dsa/.432__dsa/.432__dsa/.432__dsa/.432__dsa/.432__dsa/.432__dsa/.432__dsa/.432__dsa/.432__dsa/.432__dsa/.432__dsa/.432__dsa/.432__dsa/.432__dsa/.432__dsa/.432__dsa/.432__dsa/.432__dsa/.432__dsa/.432__dsa/.432__dsa/.432__dsa/.432__dsa/.432__dsa/.432__dsa/.432__dsa/.432__dsa/.432__dsa/.432__dsa/.432__dsa/.432__dsa/.432__dsa/.432__dsa/.432__dsa/.432__dsa/.432__dsa/.432__dsa/.432__dsa/.432__dsa/.432__dsa/.432__dsa/.432__dsa/.432__dsa/.432__dsa/.432__dsa/.432__dsa/.432__dsa/.432__dsa/.432__dsa/.432__dsa/.432__dsa/.432__dsa/.432__dsa/.432__dsa/.432__dsa/.432__dsa/.432__dsa/.432__dsa/.432__dsa/.432__dsa/.432__dsa/.432__dsa/.432__dsa/.432__dsa/.432__dsa/.432__dsa/.432__dsa/.432__dsa/.432__dsa/.432__dsa/.432__dsa/.432__dsa/.432__dsa/.432__dsa/.432__dsa/.432__dsa/.432__dsa/.432__dsa/.432__dsa/.432__dsa/.432__dsa/.432__dsa/.432__dsa/.432__dsa/.432__dsa/.432__dsa/.432__dsa/.432__dsa/.432__dsa/.432__dsa/.432__dsa/.432__dsa/.432__dsa/.432__dsa/.432__dsa/.432__dsa/.432__dsa/.432__dsa/.432__dsa/.432__dsa/.432__dsa/.432__dsa/.432__dsa/.432__dsa/.432__dsa/.432__dsa/.432__dsa/.432__dsa/.432__dsa/.432__dsa/.432__dsa/.432__dsa/.432__dsa/.432__dsa/.432__dsa/.432__dsa/.432__dsa/.432__dsa/.432__dsa/.432__dsa/.432__dsa/.432__dsa/.432__dsa/.432__dsa/.432__dsa/.432__dsa/.432__dsa/.432__dsa/.432__dsa/.432__dsa/.432__dsa/.432__dsa/.432__dsa/.432__dsa/.432__dsa/.432__dsa/.432__dsa/.432__dsa/.432__dsa/.432__dsa/.432__dsa/.432__dsa/.432__dsa/.432__dsa/.432__dsa/.432__dsa/.432__dsa/.432__dsa/.432__dsa/.432__dsa/.432__dsa/.432__dsa/.432__dsa/.432__dsa/.432__dsa/.432__dsa/.432__dsa/.432__dsa/.432__dsa/.432__dsa/.432__dsa/.432__dsa/.432__dsa/.432__dsa/.432__dsa/.432__dsa/.432__dsa/.432__dsa/.432__dsa/.432__dsa/.432__dsa/.432__dsa/.432__dsa/.432__dsa/.432__dsa/.432__dsa/.432__dsa/.432__dsa/.432__dsa/.432__dsa/.432__dsa/.432__dsa/.432__dsa/.432__dsa/.432__dsa/.432__dsa/.432__dsa/.432__dsa/.432__dsa/.432__dsa/.432__dsa/.432__dsa/.432__dsa/.432__dsa/.432__dsa/.432__dsa/.432__dsa/.432__dsa/.432__dsa/.432__dsa/.432__dsa/.432__dsa/.432__dsa/.432__dsa/.432__dsa/.432__dsa/.432__dsa/.432__dsa/.432__dsa/.432__dsa/.432__dsa/.432__dsa/.432__dsa/.432__dsa/.432__dsa/.432__dsa/.432__dsa/.432__dsa/.432__dsa/.432__dsa/.432__dsa/.432__dsa/.432__dsa/.432__dsa/.432__dsa/.432__dsa/.432__dsa/.432__dsa/.432__dsa/.432__dsa/.432__dsa/.432__dsa/.432__dsa/.432__dsa/.432__dsa/.432__dsa/.432__dsa/.432__dsa/.432__dsa/.432__dsa/.432__dsa/.432__dsa/.432__dsa/.432__dsa/.432__dsa/.432__dsa/.432__dsa/.432__dsa/.432__dsa/.432__dsa/.432__dsa/.432__dsa/.432__dsa/.432__dsa/.432__dsa/.432__dsa/.432__dsa/.432__dsa/.432__dsa/.432__dsa/.432__dsa/.432__dsa/.432__dsa/.432__dsa/.432__dsa/.432__dsa/.432__dsa/.432__dsa/.432__dsa/.432__dsa/.432__dsa/.432__dsa/.432__dsa/.432__dsa/.432__dsa/.432__dsa/.432__dsa/.432__dsa/.432__dsa/.432__dsa/.432__dsa/.432__dsa/.432__dsa/.432__dsa/.432__dsa/.432__dsa/.432__dsa/.432__dsa/.432__dsa/.432__dsa/.432__dsa/.432__dsa/.432__dsa/.432__dsa/.432__dsa/.432__dsa/.432__dsa/.432__dsa/.432__dsa/.432__dsa/.432__dsa/.432__dsa/.432__dsa/.432__dsa/.432__dsa/.432__dsa/.432__dsa/.432__dsa/.432__dsa/.432__dsa/.432__dsa/.432__dsa/.432__dsa/.432__dsa/.432__dsa/.432__dsa/.432__dsa/.432__dsa/.432__dsa/.432__dsa/.432__dsa/.432__dsa/.432__dsa/.432__dsa/.432__dsa/.432__dsa/.432__dsa/.432__dsa/.432__dsa/.432__dsa/.432__dsa/.432__dsa/.432__dsa/.432__dsa/.432__dsa/.432__dsa/.432__dsa/.432__dsa/.432__dsa/.432__dsa/.432__dsa/.432__dsa/.432__dsa/.432__dsa/.432__dsa/.432__dsa/.432__dsa/.432__dsa/.432__dsa/.432__dsa/.432__dsa/.432__dsa/.432__dsa/.432__dsa/.432__dsa/.432__dsa/.432__dsa/.432__dsa/.432__dsa/.432__dsa/.432__dsa/.432__dsa/.432__dsa/.432__dsa/.432__dsa/.432__dsa/.432__dsa/.432__dsa/.432__dsa/.432__dsa/.432__dsa/.432__dsa/.432__dsa/.432__dsa/.432__dsa/.432__dsa/.432__dsa/.432__dsa/.432__dsa/.432__dsa/.432__dsa/.432__dsa/.432__dsa/.432__dsa/.432__dsa/.432__dsa/.432__dsa/.432__dsa/.432__dsa/.432__dsa/.432__dsa/.432__dsa/.432__dsa/.432__dsa/.432__dsa/.432__dsa/.432__dsa/.432__dsa/.432__dsa/.432__dsa/.432__dsa/.432__dsa/.432__dsa/.432__dsa/.432__dsa/.432__dsa/.432__dsa/.432__dsa/.432__dsa/.432__dsa/.432__dsa/.432__dsa/.432__dsa/.432__dsa/.432__dsa/.432__dsa/.432__dsa/.432__dsa/.432__dsa/.432__dsa/.432__dsa/.432__dsa/.432__dsa/.432__dsa/.432__dsa/.432__dsa/.432__dsa/.432__dsa/.432__dsa/.432__dsa/.432__dsa/.432__dsa/.432__dsa/.432__dsa/.432__dsa/.432__dsa/.432__dsa/.432__dsa/.432__dsa/.432__dsa/.432__dsa/.432__dsa/.432__dsa/.432__dsa/.432__dsa/.432__dsa/.432__dsa/.432__dsa/.432__dsa/.432__dsa/.432__dsa/.432__dsa/.432__dsa/.432__dsa/.432__dsa/.432__dsa/.432__dsa/.432__dsa/.432__dsa/.432__dsa/.432__dsa/.432__dsa/.432__dsa/.432__dsa/.432__dsa/.432__dsa/.432__dsa/.432__dsa/.432__dsa/.432__dsa/.432__dsa/.432__dsa/.432__dsa/.432__dsa/.432__dsa/.432__dsa/.432__dsa/.432__dsa/.432__dsa/.432__dsa/.432__dsa/.432__dsa/.432__dsa/.432__dsa/.432__dsa/.432__dsa/.432__dsa/.432__dsa/.432__dsa/.432__dsa/.432__dsa/.432__dsa/.432__dsa/.432__dsa/.432__dsa/.432__dsa/.432__dsa/.432__dsa/.432__dsa/.432__dsa/.432__dsa/.432__dsa/.432__dsa/.432__dsa/.432__dsa/.432__dsa/.432__dsa/.432__dsa/.432__dsa/.432__dsa/.432__dsa/.432__dsa/.432__dsa/.432__dsa/.432__dsa/.432__dsa/.432__dsa/.432__dsa/.432__dsa/.432__dsa/.432__dsa/.432__dsa/.4ià", "$#$#$#$#$#$#$#$#$#$#$#$#$#$#$#$#$#$#$#$#$#$#$#$#$#$#$#$#$#$#$#$#$#$#$#$#$#$#$#$#$#$#$#$#$#$#$#$#$#$#$#$#$#$#$#$#$#$#$#$#$#$#$#$#$#$#$#$#$#$#$#$#$#$#$#$#$#$#$#$#$#$#$#$#$#$#$#$#$#$#$#$#$#$#$#$#$#$#$#$#$#$#$#$#$#$#$#$#$#$#$#$#$#$#$#$#$#$#$#$#$#$#$#$#$#$#$#$#$#$#$#$#$#$#$#$#$#$#$#$#$#$#$#$#$#$#$#$#$#$#$#$#$#$#$#$#$#$#$#$#$#$#$#$#$#$#$#$#$#$#$#$#$#$#$#$#$#$#$#$#$#$#$#$#$#$#$#$#$#$#$#$#$#$#$#$#$#$#$#$#$#$#$#$#$#$#$#$#$#$#$#$#$#$#$#$#$#$#$#$#$#$#$#$#$#$#$#$#$#$#$#$#$#$#$#$#$#$#$#$#$#$#$#$#$#$#$#$#$#$#$#$#$#$#$#$#$#$#$#$#$#$#$#$#$#$#$#$#$#$#$#$#$#$#$#$#$#$#$#$#$#$#$#$#$#$#$#$#$#$#$#$#$#$#$#$#$#$#$#$#$#$#$#$#$#$#$#$#$#$#$#$#$#$#$#$#$#$#$#$#$#$#$#$#$#$#$#$#$#$#$#$#$#$#$#$#$#$#$#$#$#$#$#$#$#$#$#$#$#$#$#$#$#$#$#$#$#$#$#$#$#$#$#$#$#$#$#$#$#$#$#$#$#$#$#$#$#$#$#$#$#$#$#$#$#$#$#$#$#$#$#$#$#$#$#$#$#$#$#$#$#$#$#$#$#$#$#$#$#$#$#$#$#$#$#$#$#$#$#$#$#$#$#$#$#$#$#$#$#$#$#$#$#$#$#$#$#$#$#$#$#$#$#$#$#$#$#$#$#$#$#$#$#$#$#$#$#$#$#$#$#$#$#$#$#$#$#$#$#$#$#$#$#$#$#$#$#$#$#$#$#$#$#$#$#$#$#$#$#$#$#$#$#$#$#$#$#$#$#$#$#$#$#$#$#$#$#$#$#$#$#$#$#$#$#$#$#$#$#$#$#$#$#$#$#$#$#$#$#$#$#$#$#$#$#$#$#$#$#$#$#$#$#$#$#$#$#$#$#$#$#$#$#$#$#$#$#$#$#$#$#$#$#$#$#$#$#$#$#$#$#$#$#$#$#$#$#$#$#$#$#$#$#$#$#$#$#$#$#$#$#$#$#$#$#$#$#$#$#$#$#$#$#$#$#$#$#$#$#$#$#$#$#$#$#$#$#$#$#$#$#$#$#$#$#$#$#$#$#$#$#$#$#$#$#$#$#$#$#$#$#$#$#$#$#$#$#$#$#$#$#$#$#$#$#$#$#$#$#$#$#$#$#$#$#$#$#$#$#$#$#$#$#$#$#$#$#$#$#$#$#$#$#$#$#$#$#$#$#$#$#$#$#$#$#$#$#$#$#$#$#$#$#$#$#$#$#$#$#$#$#$#$#$#$#$#$#$#$#$#$#$#$#$#$#$#$#$#$#$#$#$#$#$#$#$#$#$#$#$#$#$#$#$#$#$#$#$#$#$#$#$#$#$#$#$#$#$#$#$#$#$#$#$#$#$#$#$#$#$#$#$#$#$#$#$#$#$#$#$#$#$#$#$#$#$#$#$#$#$#$#$#$#$#$#$#$#$#$#$#$#$#$#$#$#$#$#$#$#$#$#$#$#$#$#$#$#$#$#$#$#$#$#$#$#$#$#$#$#$#$#$#$#$#$#$#$#$#$#$#$#$#$#$#$#$#$#$#$#$#$#$#$#$#$#$#$#$#$#$#$#$#$#$#$#$#$#$#$#$#$#$#$#$#$#$#$#$#$#$#$#$#$#$#$#$#$#$#$#$#$#$#$#$#$#$#$#$#$#$#$#$#$#$#$#$#$#$#$#$#$#$#$#$#$#$#$#$#$#$#$#$#$#$#$#$#$#$#$#$#$#$#$#$#$#$#$#$#$#$#$#$#$#$#$#$#$#$#$#$#$#$#$#$#$#$#$#$#$#$#$#$#$#$#$#$#$#$#$#$#$#$#$#$#$#$#$#$#$#$#$#$#$#$#$#$#$#$#$#$#$#$#$#$#$#$#$#$#$#\u0015X", "pjlt';\\]`pjlt';\\]`pjlt';\\]`pjlt';\\]`pjlt';\\]`pjlt';\\]`pjlt';\\]`pjlt';\\]`pjlt';\\]`pjlt';\\]`pjlt';\\]`pjlt';\\]`pjlt';\\]`pjlt';\\]`pjlt';\\]`pjlt';\\]`pjlt';\\]`pjlt';\\]`pjlt';\\]`pjlt';\\]`pjlt';\\]`pjlt';\\]`pjlt';\\]`pjlt';\\]`pjlt';\\]`pjlt';\\]`pjlt';\\]`pjlt';\\]`pjlt';\\]`pjlt';\\]`pjlt';\\]`pjlt';\\]`pjlt';\\]`pjlt';\\]`pjlt';\\]`pjlt';\\]`pjlt';\\]`pjlt';\\]`pjlt';\\]`pjlt';\\]`pjlt';\\]`pjlt';\\]`pjlt';\\]`pjlt';\\]`pjlt';\\]`pjlt';\\]`pjlt';\\]`pjlt';\\]`pjlt';\\]`pjlt';\\]`pjlt';\\]`pjlt';\\]`pjlt';\\]`pjlt';\\]`pjlt';\\]`pjlt';\\]`pjlt';\\]`pjlt';\\]`pjlt';\\]`pjlt';\\]`pjlt';\\]`pjlt';\\]`pjlt';\\]`pjlt';\\]`pjlt';\\]`pjlt';\\]`pjlt';\\]`pjlt';\\]`pjlt';\\]`pjlt';\\]`pjlt';\\]`pjlt';\\]`pjlt';\\]`pjlt';\\]`pjlt';\\]`pjlt';\\]`pjlt';\\]`pjlt';\\]`pjlt';\\]`pjlt';\\]`pjlt';\\]`pjlt';\\]`pjlt';\\]`pjlt';\\]`pjlt';\\]`pjlt';\\]`pjlt';\\]`pjlt';\\]`pjlt';\\]`pjlt';\\]`pjlt';\\]`pjlt';\\]`pjlt';\\]`pjlt';\\]`pjlt';\\]`pjlt';\\]`pjlt';\\]`pjlt';\\]`pjlt';\\]`pjlt';\\]`pjlt';\\]`pjlt';\\]`pjlt';\\]`pjlt';\\]`pjlt';\\]`pjlt';\\]`pjlt';\\]`pjlt';\\]`pjlt';\\]`pjlt';\\]`pjlt';\\]`pjlt';\\]`pjlt';\\]`pjlt';\\]`pjlt';\\]`pjlt';\\]`pjlt';\\]`pjlt';\\]`pjlt';\\]`pjlt';\\]`pjlt';\\]`pjlt';\\]`pjlt';\\]`pjlt';\\]`pjlt';\\]`pjlt';\\]`pjlt';\\]`pjlt';\\]`pjlt';\\]`pjlt';\\]`pjlt';\\]`pjlt';\\]`pjlt';\\]`pjlt';\\]`pjlt';\\]`pjlt';\\]`pjlt';\\]`pjlt';\\]`pjlt';\\]`pjlt';\\]`pjlt';\\]`pjlt';\\]`pjlt';\\]`pjlt';\\]`pjlt';\\]`pjlt';\\]`pjlt';\\]`pjlt';\\]`pjlt';\\]`pjlt';\\]`pjlt';\\]`pjlt';\\]`pjlt';\\]`pjlt';\\]`pjlt';\\]`pjlt';\\]`pjlt';\\]`pjlt';\\]`pjlt';\\]`pjlt';\\]`pjlt';\\]`pjlt';\\]`pjlt';\\]`pjlt';\\]`pjlt';\\]`pjlt';\\]`pjlt';\\]`pjlt';\\]`pjlt';\\]`pjlt';\\]`pjlt';\\]`pjlt';\\]`pjlt';\\]`pjlt';\\]`pjlt';\\]`pjlt';\\]`pjlt';\\]`pjlt';\\]`pjlt';\\]`pjlt';\\]`pjlt';\\]`pjlt';\\]`pjlt';\\]`pjlt';\\]`pjlt';\\]`pjlt';\\]`pjlt';\\]`pjlt';\\]`pjlt';\\]`pjlt';\\]`pjlt';\\]`pjlt';\\]`pjlt';\\]`pjlt';\\]`pjlt';\\]`pjlt';\\]`pjlt';\\]`pjlt';\\]`pjlt';\\]`pjlt';\\]`pjlt';\\]`pjlt';\\]`pjlt';\\]`pjlt';\\]`pjlt';\\]`pjlt';\\]`pjlt';\\]`pjlt';\\]`pjlt';\\]`pjlt';\\]`pjlt';\\]`pjlt';\\]`pjlt';\\]`pjlt';\\]`pjlt';\\]`pjlt';\\]`pjlt';\\]`pjlt';\\]`pjlt';\\]`pjlt';\\]`pjlt';\\]`pjlt';\\]`pjlt';\\]`pjlt';\\]`pjlt';\\]`pjlt';\\]`pjlt';\\]`pjlt';\\]`pjlt';\\]`pjlt';\\]`pjlt';\\]`pjlt';\\]`pjlt';\\]`pjlt';\\]`pjlt';\\]`pjlt';\\]`pjlt';\\]`pjlt';\\]`pjlt';\\]`pjlt';\\]`pjlt';\\]`pjlt';\\]`pjlt';\\]`pjlt';\\]`pjlt';\\]`pjlt';\\]`pjlt';\\]`pjlt';\\]`pjlt';\\]`pjlt';\\]`pjlt';\\]`pjlt';\\]`pjlt';\\]`pjlt';\\]`pjlt';\\]`pjlt';\\]`pjlt';\\]`pjlt';\\]`pjlt';\\]`pjlt';\\]`pjlt';\\]`pjlt';\\]`pjlt';\\]`pjlt';\\]`pjlt';\\]`pjlt';\\]`pjlt';\\]`pjlt';\\]`pjlt';\\]`pjlt';\\]`pjlt';\\]`pjlt';\\]`pjlt';\\]`pjlt';\\]`pjlt';\\]`pjlt';\\]`pjlt';\\]`pjlt';\\]`pjlt';\\]`pjlt';\\]`pjlt';\\]`pjlt';\\]`pjlt';\\]`pjlt';\\]`pjlt';\\]`pjlt';\\]`pjlt';\\]`pjlt';\\]`pjlt';\\]`pjlt';\\]`pjlt';\\]`pjlt';\\]`pjlt';\\]`pjlt';\\]`pjlt';\\]`pjlt';\\]`pjlt';\\]`pjlt';\\]`pjlt';\\]`pjlt';\\]`pjlt';\\]`pjlt';\\]`pjlt';\\]`pjlt';\\]`pjlt';\\]`pjlt';\\]`pjlt';\\]`pjlt';\\]`pjlt';\\]`pjlt';\\]`pjlt';\\]`pjlt';\\]`pjlt';\\]`pjlt';\\]`pjlt';\\]`pjlt';\\]`pjlt';\\]`pjlt';\\]`pjlt';\\]`pjlt';\\]`pjlt';\\]`pjlt';\\]`pjlt';\\]`pjlt';\\]`pjlt';\\]`pjlt';\\]`pjlt';\\]`pjlt';\\]`pjlt';\\]`pjlt';\\]`pjlt';\\]`pjlt';\\]`pjlt';\\]`pjlt';\\]`pjlt';\\]`pjlt';\\]`pjlt';\\]`pjlt';\\]`pjlt';\\]`pjlt';\\]`pjlt';\\]`pjlt';\\]`pjlt';\\]`pjlt';\\]`pjlt';\\]`pjlt';\\]`pjlt';\\]`pjlt';\\]`pjlt';\\]`pjlt';\\]`pjlt';\\]`pjlt';\\]`pjlt';\\]`pjlt';\\]`pjlt';\\]`pjlt';\\]`pjlt';\\]`pjlt';\\]`pjlt';\\]`pjlt';\\]`pjlt';\\]`pjlt';\\]`pjlt';\\]`pjlt';\\]`pjlt';\\]`pjlt';\\]`pjlt';\\]`pjlt';\\]`pjlt';\\]`pjlt';\\]`pjlt';\\]`pjlt';\\]`pjlt';\\]`pjlt';\\]`pjlt';\\]`pjlt';\\]`pjlt';\\]`pjlt';\\]`pjlt';\\]`pjlt';\\]`pjlt';\\]`pjlt';\\]`pjlt';\\]`pjlt';\\]`pjlt';\\]`pjlt';\\]`pjlt';\\]`pjlt';\\]`pjlt';\\]`pjlt';\\]`pjlt';\\]`pjlt';\\]`pjlt';\\]`pjlt';\\]`pjlt';\\]`pjlt';\\]`pjlt';\\]`pjlt';\\]`pjlt';\\]`pjlt';\\]`pjlt';\\]`pjlt';\\]`pjlt';\\]`pjlt';\\]`pjlt';\\]`pjlt';\\]`pjlt';\\]`pjlt';\\]`pjlt';\\]`pjlt';\\]`pjlt';\\]`pjlt';\\]`pjlt';\\]`pjlt';\\]`pjlt';\\]`pjlt';\\]`pjlt';\\]`pjlt';\\]`pjlt';\\]`pjlt';\\]`pjlt';\\]`pjlt';\\]`pjlt';\\]`pjlt';\\]`pjlt';\\]`pjlt';\\]`pjlt';\\]`pjlt';\\]`pjlt';\\]`pjlt';\\]`pjlt';\\]`pjlt';\\]`pjlt';\\]`pjlt';\\]`pjlt';\\]`pjlt';\\]`pjlt';\\]`pjlt';\\]`pjlt';\\]`pjlt';\\]`pjlt';\\]`pjlt';\\]`pjlt';\\]`pjlt';\\]`pjlt';\\]`pjlt';\\]`pjlt';\\]`pjlt';\\]`pjlt';\\]`pjlt';\\]`pjlt';\\]`pjlt';\\]`pjlt';\\]`pjlt';\\]`pjlt';\\]`pjlt';\\]`pjlt';\\]`pjlt';\\]`pjlt';\\]`pjlt';\\]`pjlt';\\]`pjlt';\\]`pjlt';\\]`pjlt';\\]`pjlt';\\]`pjlt';\\]`pjlt';\\]`pjlt';\\]`pjlt';\\]`pjlt';\\]`pjlt';\\]`pjlt';\\]`pjlt';\\]`pjlt';\\]`pjlt';\\]`pjlt';\\]`pjlt';\\]`pjlt';\\]`pjlt';\\]`pjlt';\\]`pjlt';\\]`pjlt';\\]`pjlt';\\]`pjlt';\\]`pjlt';\\]`pjlt';\\]`pjlt';\\]`pjlt';\\]`pjlt';\\]`pjlt';\\]`pjlt';\\]`pjlt';\\]`pjlt';\\]`pjlt';\\]`pjlt';\\]`pjlt';\\]`pjlt';\\]`pjlt';\\]`pjlt';\\]`pjlt';\\]`pjlt';\\]`pjlt';\\]`pjlt';\\]`pjlt';\\]`pjlt';\\]`pjlt';\\]`pjlt';\\]`pjlt';\\]`pjlt';\\]`pjlt';\\]`pjlt';\\]`pjlt';\\]`pjlt';\\]`pjlt';\\]`pjlt';\\]`pjlt';\\]`pjlt';\\]`pjlt';\\]`pjlt';\\]`pjlt';\\]`pjlt';\\]`pjlt';\\]`pjlt';\\]`pjlt';\\]`pjlt';\\]`pjlt';\\]`pjlt';\\]`pjlt';\\]`pjlt';\\]`pjlt';\\]`pjlt';\\]`pjlt';\\]`pjlt';\\]`pjlt';\\]`pjlt';\\]`pjlt';\\]`pjlt';\\]`pjlt';\\]`pjlt';\\]`pjlt';\\]`pjlt';\\]`pjlt';\\]`pjlt';\\]`pjlt';\\]`pjlt';\\]`pjlt';\\]`pjlt';\\]`pjlt';\\]`pjlt';\\]`pjlt';\\]`pjlt';\\]`pjlt';\\]`pjlt';\\]`pjlt';\\]`pjlt';\\]`pjlt';\\]`pjlt';\\]`pjlt';\\]`pjlt';\\]`pjlt';\\]`pjlt';\\]`pjlt';\\]`pjlt';\\]`pjlt';\\]`pjlt';\\]`pjlt';\\]`pjlt';\\]`pjlt';\\]`pjlt';\\]`pjlt';\\]`pjlt';\\]`pjlt';\\]`pjlt';\\]`pjlt';\\]`pjlt';\\]`pjlt';\\]`pjlt';\\]`pjlt';\\]`pjlt';\\]`pjlt';\\]`pjlt';\\]`pjlt';\\]`pjlt';\\]`pjlt';\\]`pjlt';\\]`pjlt';\\]`pjlt';\\]`pjlt';\\]`pjlt';\\]`pjlt';\\]`pjlt';\\]`pjlt';\\]`pjlt';\\]`pjlt';\\]`pjlt';\\]`pjlt';\\]`pjlt';\\]`pjlt';\\]`pjlt';\\]`pjlt';\\]`pjlt';\\]`pjlt';\\]`pjlt';\\]`pjlt';\\]`pjlt';\\]`pjlt';\\]`pjlt';\\]`pjlt';\\]`pjlt';\\]`pjlt';\\]`pjlt';\\]`pjlt';\\]`pjlt';\\]`pjlt';\\]`pjlt';\\]`pjlt';\\]`pjlt';\\]`pjlt';\\]`pjlt';\\]`pjlt';\\]`pjlt';\\]`pjlt';\\]`pjlt';\\]`pjlt';\\]`pjlt';\\]`pjlt';\\]`pjlt';\\]`pjlt';\\]`pjlt';\\]`pjlt';\\]`pjlt';\\]`pjlt';\\]`pjlt';\\]`pjlt';\\]`pjlt';\\]`pjlt';\\]`pjlt';\\]`pjlt';\\]`pjlt';\\]`pjlt';\\]`pjlt';\\]`pjlt';\\]`pjlt';\\]`pjlt';\\]`pjlt';\\]`pjlt';\\]`pjlt';\\]`pjlt';\\]`pjlt';\\]`pjlt';\\]`pjlt';\\]`pjlt';\\]`pjlt';\\]`pjlt';\\]`pjlt';\\]`pjlt';\\]`pjlt';\\]`pjlt';\\]`pjlt';\\]`pjlt';\\]`pjlt';\\]`pjlt';\\]`pjlt';\\]`pjlt';\\]`pjlt';\\]`pjlt';\\]`pjlt';\\]`pjlt';\\]`pjlt';\\]`pjlt';\\]`pjlt';\\]`pjlt';\\]`pjlt';\\]`pjlt';\\]`pjlt';\\]`pjlt';\\]`pjlt';\\]`pjlt';\\]`pjlt';\\]`pjlt';\\]`pjlt';\\]`pjlt';\\]`pjlt';\\]`pjlt';\\]`pjlt';\\]`pjlt';\\]`pjlt';\\]`pjlt';\\]`pjlt';\\]`pjlt';\\]`pjlt';\\]`pjlt';\\]`pjlt';\\]`pjlt';\\]`pjlt';\\]`pjlt';\\]`pjlt';\\]`pjlt';\\]`pjlt';\\]`pjlt';\\]`pjlt';\\]`pjlt';\\]`pjlt';\\]`pjlt';\\]`pjlt';\\]`pjlt';\\]`pjlt';\\]`pjlt';\\]`pjlt';\\]`pjlt';\\]`pjlt';\\]`pjlt';\\]`pjlt';\\]`pjlt';\\]`pjlt';\\]`pjlt';\\]`pjlt';\\]`pjlt';\\]`pjlt';\\]`pjlt';\\]`pjlt';\\]`pjlt';\\]`pjlt';\\]`pjlt';\\]`pjlt';\\]`pjlt';\\]`pjlt';\\]`pjlt';\\]`pjlt';\\]`pjlt';\\]`pjlt';\\]`pjlt';\\]`pjlt';\\]`pjlt';\\]`pjlt';\\]`pjlt';\\]`pjlt';\\]`pjlt';\\]`pjlt';\\]`pjlt';\\]`pjlt';\\]`pjlt';\\]`pjlt';\\]`pjlt';\\]`pjlt';\\]`pjlt';\\]`pjlt';\\]`pjlt';\\]`pjlt';\\]`pjlt';\\]`pjlt';\\]`pjlt';\\]`pjlt';\\]`pjlt';\\]`pjlt';\\]`pjlt';\\]`pjlt';\\]`pjlt';\\]`pjlt';\\]`pjlt';\\]`pjlt';\\]`pjlt';\\]`pjlt';\\]`pjlt';\\]`pjlt';\\]`pjlt';\\]`pjlt';\\]`pjlt';\\]`pjlt';\\]`pjlt';\\]`pjlt';\\]`pjlt';\\]`pjlt';\\]`pjlt';\\]`pjlt';\\]`pjlt';\\]`pjlt';\\]`pjlt';\\]`pjlt';\\]`pjlt';\\]`pjlt';\\]`pjlt';\\]`pjlt';\\]`pjlt';\\]`pjlt';\\]`pjlt';\\]`pjlt';\\]`pjlt';\\]`pjlt';\\]`pjlt';\\]`pjlt';\\]`pjlt';\\]`pjlt';\\]`pjlt';\\]`pjlt';\\]`pjlt';\\]`pjlt';\\]`pjlt';\\]`pjlt';\\]`pjlt';\\]`pjlt';\\]`pjlt';\\]`pjlt';\\]`pjlt';\\]`pjlt';\\]`pjlt';\\]`pjlt';\\]`pjlt';\\]`pjlt';\\]`pjlt';\\]`pjlt';\\]`pjlt';\\]`pjlt';\\]`pjlt';\\]`pjlt';\\]`pjlt';\\]`pjlt';\\]`pjlt';\\]`pjlt';\\]`pjlt';\\]`pjlt';\\]`pjlt';\\]`pjlt';\\]`pjlt';\\]`pjlt';\\]`pjlt';\\]`pjlt';\\]`pjlt';\\]`pjlt';\\]`pjlt';\\]`pjlt';\\]`pjlt';\\]`pjlt';\\]`pjlt';\\]`pjlt';\\]`pjlt';\\]`pjlt';\\]`pjlt';\\]`pjlt';\\]`pjlt';\\]`pjlt';\\]`pjlt';\\]`pjlt';\\]`pjlt';\\]`pjlt';\\]`pjlt';\\]`pjlt';\\]`pjlt';\\]`pjlt';\\]`pjlt';\\]`pjlt';\\]`pjlt';\\]`pjlt';\\]`pjlt';\\]`pjlt';\\]`pjlt';\\]`pjlt';\\]`pjlt';\\]`pjlt';\\]`pjlt';\\]`pjlt';\\]`pjlt';\\]`pjlt';\\]`pjlt';\\]`pjlt';\\]`pjlt';\\]`pjlt';\\]`pjlt';\\]`pjlt';\\]`pjlt';\\]`pjlt';\\]`pjlt';\\]`pjlt';\\]`pjlt';\\]`pjlt';\\]`pjlt';\\]`pjlt';\\]`pjlt';\\]`pjlt';\\]`pjlt';\\]`pjlt';\\]`pjlt';\\]`pjlt';\\]`pjlt';\\]`pjlt';\\]`pjlt';\\]`pjlt';\\]`pjlt';\\]`pjlt';\\]`pjlt';\\]`pjlt';\\]`pjlt';\\]`pjlt';\\]`pjlt';\\]`pjlt';\\]`pjlt';\\]`pjlt';\\]`pjlt';\\]`pjlt';\\]`pjlt';\\]`pjlt';\\]`pjlt';\\]`pjlt';\\]`pjlt';\\]`pjlt';\\]`pjlt';\\]`pjlt';\\]`pjlt';\\]`pjlt';\\]`pjlt';\\]`pjlt';\\]`pjlt';\\]`pjlt';\\]`pjlt';\\]`pjlt';\\]`pjlt';\\]`pjlt';\\]`pjlt';\\]`pjlt';\\]`pjlt';\\]`pjlt';\\]`pjlt';\\]`pjlt';\\]`pjlt';\\]`pjlt';\\]`pjlt';\\]`pjlt';\\]`pjlt';\\]`pjlt';\\]`pjlt';\\]`pjlt';\\]`pjlt';\\]`pjlt';\\]`pjlt';\\]`pjlt';\\]`pjlt';\\]`pjlt';\\]`pjlt';\\]`pjlt';\\]`pjlt';\\]`pjlt';\\]`pjlt';\\]`pjlt';\\]`pjlt';\\]`pjlt';\\]`pjlt';\\]`pjlt';\\]`pjlt';\\]`pjlt';\\]`pjlt';\\]`pjlt';\\]`pjlt';\\]`pjlt';\\]`pjlt';\\]`pjlt';\\]`pjlt';\\]`pjlt';\\]`pjlt';\\]`pjlt';\\]`pjlt';\\]`pjlt';\\]`pjlt';\\]`pjlt';\\]`pjlt';\\]`pjlt';\\]`pjlt';\\]`pjlt';\\]`pjlt';\\]`pjlt';\\]`pjlt';\\]`pjlt';\\]`pjlt';\\]`pjlt';\\]`pjlt';\\]`pjlt';\\]`pjlt';\\]`pjlt';\\]`pjlt';\\]`pjlt';\\]`pjlt';\\]`pjlt';\\]`pjlt';\\]`pjlt';\\]`pjlt';\\]`pjlt';\\]`pjlt';\\]`pjlt';\\]`pjlt';\\]`pjlt';\\]`pjlt';\\]`pjlt';\\]`pjlt';\\]`pjlt';\\]`pjlt';\\]`pjlt';\\]`pjlt';\\]`pjlt';\\]`pjlt';\\]`pjlt';\\]`pjlt';\\‡\b", "~~~~~~~~~~~~~~~~~~~~~~~~~~~~~~~~~~~~~~~~~~~~~~~~~~~~~~~~~~~~~~~~~~~~~~~~~~~~~~~~~~~~~~~~~~~~~~~~~~~~~~~~~~~~~~~~~~~~~~~~~~~~~~~~~~~~~~~~~~~~~~~~~~~~~~~~~~~~~~~~~~~~~~~~~~~~~~~~~~~~~~~~~~~~~~~~~~~~~~~~~~~~~~~~~~~~~~~~~~~~~~~~~~~~~~~~~~~~~~~~~~~~~~~~~~~~~~~~~~~~~~~~~~~~~~~~~~~~~~~~~~~~~~~~~~~~~~~~~~~~~~~~~~~~~~~~~~~~~~~~~~~~~~~~~~~~~~~~~~~~~~~~~~~~~~~~~~~~~~~~~~~~~~~~~~~~~~~~~~~~~~~~~~~~~~~~~~~~~~~~~~~~~~~~~~~~~~~~~~~~~~~~~~~~~~~~~~~~~~~~~~~~~~~~~~~~~~~~~~~~~~~~~~~~~~~~~~~~~~~~~~~~~~~~~~~~~~~~~~~~~~~~~~~~~~~~~~~~~~~~~~~~~~~~~~~~~~~~~~~~~~~~~~~~~~~~~~~~~~~~~~~~~~~~~~~~~~~~~~~~~~~~~~~~~~~~~~~~~~~~~~~~~~~~~~~~~~~~~~~~~~~~~~~~~~~~~~~~~~~~~~~~~~~~~~~~~~~~~~~~~~~~~~~~~~~~~~~~~~~~~~~~~~~~~~~~~~~~~~~~~~~~~~~~~~~~~~~~~~~~~~~~~~~~~~~~~~~~~~~~~~~~~~~~~~~~~~~~~~~~~~~~~~~~~~~~~~~~~~~~~~~~~~~~~~~~~~~~~~~~~~~~~~~~~~~~~~~~~~~~~~~~~~~~~~~~~~~~~~~~~~~~~~~~~~~~~~~~~~~~~~~~~~~~~~~~~~~~~~~~~~~~~~~~~~~~~~~~~~~~~~~~~~~~~~~~~~~~~~~~~~~~~~~~~~~~~~~~~~~~~~~~~~~~~~~~~~~~~~~~~~~~~~~~~~~~~~~~~~~~~~~~~~~~~~~~~~~~~~ì0", "LabVIEWLabVIEWLabVIEWLabVIEWLabVIEWLabVIEWLabVIEWLabVIEWLabVIEWLabVIEWLabVIEWLabVIEWLabVIEWLabVIEWLabVIEWLabVIEWLabVIEWLabVIEWLabVIEWLabVIEWLabVIEWLabVIEWLabVIEWLabVIEWLabVIEWLabVIEWLabVIEWLabVIEWLabVIEWLabVIEWLabVIEWLabVIEWLabVIEWLabVIEWLabVIEWLabVIEWLabVIEWLabVIEWLabVIEWLabVIEWLabVIEWLabVIEWLabVIEWLabVIEWLabVIEWLabVIEWLabVIEWLabVIEWLabVIEWLabVIEWLabVIEWLabVIEWLabVIEWLabVIEWLabVIEWLabVIEWLabVIEWLabVIEWLabVIEWLabVIEWLabVIEWLabVIEWLabVIEWLabVIEWLabVIEWLabVIEWLabVIEWLabVIEWLabVIEWLabVIEWLabVIEWLabVIEWLabVIEWLabVIEWLabVIEWLabVIEWLabVIEWLabVIEWLabVIEWLabVIEWLabVIEWLabVIEWLabVIEWLabVIEWLabVIEWLabVIEWLabVIEWLabVIEWLabVIEWLabVIEWLabVIEWLabVIEWLabVIEWLabVIEWLabVIEWLabVIEWLabVIEWLabVIEWLabVIEWLabVIEWLabVIEWLabVIEWLabVIEWLabVIEWLabVIEWLabVIEWLabVIEWLabVIEWLabVIEWLabVIEWLabVIEWLabVIEWLabVIEWLabVIEWLabVIEWLabVIEWLabVIEWLabVIEWLabVIEWLabVIEWLabVIEWLabVIEWLabVIEWLabVIEWLabVIEWLabVIEWLabVIEWLabVIEWLabVIEWLabVIEWLabVIEWLabVIEWLabVIEWLabVIEWLabVIEWLabVIEWLabVIEWLabVIEWLabVIEWLabVIEWLabVIEWLabVIEWLabVIEWLabVIEWLabVIEWLabVIEWLabVIEWLabVIEWLabVIEWLabVIEWLabVIEWLabVIEWLabVIEWLabVIEWLabVIEWLabVIEWLabVIEWLabVIEWLabVIEWLabVIEWLabVIEWLabVIEWLabVIEWLabVIEWLabVIEWLabVIEWLabVIEWLabVIEWLabVIEWLabVIEWLabVIEWLabVIEWLabVIEWLabVIEWLabVIEWLabVIEWLabVIEWLabVIEWLabVIEWLabVIEWLabVIEWLabVIEWLabVIEWLabVIEWLabVIEWLabVIEWLabVIEWLabVIEWLabVIEWLabVIEWLabVIEWLabVIEWLabVIEWLabVIEWLabVIEWLabVIEWLabVIEWLabVIEWLabVIEWLabVIEWLabVIEWLabVIEWLabVIEWLabVIEWLabVIEWLabVIEWLabVIEWLabVIEWLabVIEWLabVIEWLabVIEWLabVIEWLabVIEWLabVIEWLabVIEWLabVIEWLabVIEWLabVIEWLabVIEWLabVIEWLabVIEWLabVIEWLabVIEWLabVIEWLabVIEWLabVIEWLabVIEWLabVIEWLabVIEWLabVIEWLabVIEWLabVIEWLabVIEWLabVIEWLabVIEWLabVIEWLabVIEWLabVIEWLabVIEWLabVIEWLabVIEWLabVIEWLabVIEWLabVIEWLabVIEWLabVIEWLabVIEWLabVIEWLabVIEWLabVIEWLabVIEWLabVIEWLabVIEWLabVIEWLabVIEWLabVIEWLabVIEWLabVIEWLabVIEWLabVIEWLabVIEWLabVIEWLabVIEWLabVIEWLabVIEWLabVIEWLabVIEWLabVIEWLabVIEWLabVIEWLabVIEWLabVIEWLabVIEWLabVIEWLabVIEWLabVIEWLabVIEWLabVIEWLabVIEWLabVIEWLabVIEWLabVIEWLabVIEWLabVIEWLabVIEWLabVIEWLabVIEWLabVIEWLabVIEWLabVIEWLabVIEWLabVIEWLabVIEWLabVIEWLabVIEWLabVIEWLabVIEWLabVIEWLabVIEWLabVIEWLabVIEWLabVIEWLabVIEWLabVIEWLabVIEWLabVIEWLabVIEWLabVIEWLabVIEWLabVIEWLabVIEWLabVIEWLabVIEWLabVIEWLabVIEWLabVIEWLabVIEWLabVIEWLabVIEWLabVIEWLabVIEWLabVIEWLabVIEWLabVIEWLabVIEWLabVIEWLabVIEWLabVIEWLabVIEWLabVIEWLabVIEWLabVIEWLabVIEWLabVIEWLabVIEWLabVIEWLabVIEWLabVIEWLabVIEWLabVIEWLabVIEWLabVIEWLabVIEWLabVIEWLabVIEWLabVIEWLabVIEWLabVIEWLabVIEWLabVIEWLabVIEWLabVIEWLabVIEWLabVIEWLabVIEWLabVIEWLabVIEWLabVIEWLabVIEWLabVIEWLabVIEWLabVIEWLabVIEWLabVIEWLabVIEWLabVIEWLabVIEWLabVIEWLabVIEWLabVIEWLabVIEWLabVIEWLabVIEWLabVIEWLabVIEWLabVIEWLabVIEWLabVIEWLabVIEWLabVIEWLabVIEWLabVIEWLabVIEWLabVIEWLabVIEWLabVIEWLabVIEWLabVIEWLabVIEWLabVIEWLabVIEWLabVIEWLabVIEWLabVIEWLabVIEWLabVIEWLabVIEWLabVIEWLabVIEWLabVIEWLabVIEWLabVIEWLabVIEWLabVIEWLabVIEWLabVIEWLabVIEWLabVIEWLabVIEWLabVIEWLabVIEWLabVIEWLabVIEWLabVIEWLabVIEWLabVIEWLabVIEWLabVIEWLabVIEWLabVIEWLabVIEWLabVIEWLabVIEWLabVIEWLabVIEWLabVIEWLabVIEWLabVIEWLabVIEWLabVIEWLabVIEWLabVIEWLabVIEWLabVIEWLabVIEWLabVIEWLabVIEWLabVIEWLabVIEWLabVIEWLabVIEWLabVIEWLabVIEWLabVIEWLabVIEWLabVIEWLabVIEWLabVIEWLabVIEWLabVIEWLabVIEWLabVIEWLabVIEWLabVIEWLabVIEWLabVIEWLabVIEWLabVIEWLabVIEWLabVIEWLabVIEWLabVIEWLabVIEWLabVIEWLabVIEWLabVIEWLabVIEWLabVIEWLabVIEWLabVIEWLabVIEWLabVIEWLabVIEWLabVIEWLabVIEWLabVIEWLabVIEWLabVIEWLabVIEWLabVIEWLabVIEWLabVIEWLabVIEWLabVIEWLabVIEWLabVIEWLabVIEWLabVIEWLabVIEWLabVIEWLabVIEWLabVIEWLabVIEWLabVIEWLabVIEWLabVIEWLabVIEWLabVIEWLabVIEWLabVIEWLabVIEWLabVIEWLabVIEWLabVIEWLabVIEWLabVIEWLabVIEWLabVIEWLabVIEWLabVIEWLabVIEWLabVIEWLabVIEWLabVIEWLabVIEWLabVIEWLabVIEWLabVIEWLabVIEWLabVIEWLabVIEWLabVIEWLabVIEWLabVIEWLabVIEWLabVIEWLabVIEWLabVIEWLabVIEWLabVIEWLabVIEWLabVIEWLabVIEWLabVIEWLabVIEWLabVIEWLabVIEWLabVIEWLabVIEWLabVIEWLabVIEWLabVIEWLabVIEWLabVIEWLabVIEWLabVIEWLabVIEWLabVIEWLabVIEWLabVIEWLabVIEWLabVIEWLabVIEWLabVIEWLabVIEWLabVIEWLabVIEWLabVIEWLabVIEWLabVIEWLabVIEWLabVIEWLabVIEWLabVIEWLabVIEWLabVIEWLabVIEWLabVIEWLabVIEWLabVIEWLabVIEWLabVIEWLabVIEWLabVIEWLabVIEWLabVIEWLabVIEWLabVIEWLabVIEWLabVIEWLabVIEWLabVIEWLabVIEWLabVIEWLabVIEWLabVIEWLabVIEWLabVIEWLabVIEWLabVIEWLabVIEWLabVIEWLabVIEWLabVIEWLabVIEWLabVIEWLabVIEWLabVIEWLabVIEWLabVIEWLabVIEWLabVIEWLabVIEWLabVIEWLabVIEWLabVIEWLabVIEWLabVIEWLabVIEWLabVIEWLabVIEWLabVIEWLabVIEWLabVIEWLabVIEWLabVIEWLabVIEWLabVIEWLabVIEWLabVIEWLabVIEWLabVIEWLabVIEWLabVIEWLabVIEWLabVIEWLabVIEWLabVIEWLabVIEWLabVIEWLabVIEWLabVIEWLabVIEWLabVIEWLabVIEWLabVIEWLabVIEWLabVIEWLabVIEWLabVIEWLabVIEWLabVIEWLabVIEWLabVIEWLabVIEWLabVIEWLabVIEWLabVIEWLabVIEWLabVIEWLabVIEWLabVIEWLabVIEWLabVIEWLabVIEWLabVIEWLabVIEWLabVIEWLabVIEWLabVIEWLabVIEWLabVIEWLabVIEWLabVIEWLabVIEWLabVIEWLabVIEWLabVIEWLabVIEWLabVIEWLabVIEWLabVIEWLabVIEWLabVIEWLabVIEWLabVIEWLabVIEWLabVIEWLabVIEWLabVIEWLabVIEWLabVIEWLabVIEWLabVIEWLabVIEWLabVIEWLabVIEWLabVIEWLabVIEWLabVIEWLabVIEWLabVIEWLabVIEWLabVIEWLabVIEWLabVIEWLabVIEWLabVIEWLabVIEWLabVIEWLabVIEWLabVIEWLabVIEWLabVIEWLabVIEWLabVIEWLabVIEWLabVIEWLabVIEWLabVIEWLabVIEWLabVIEWLabVIEWLabVIEWLabVIEWLabVIEWLabVIEWLabVIEWLabVIEWLabVIEWLabVIEWLabVIEWLabVIEWLabVIEWLabVIEWLabVIEWLabVIEWLabVIEWLabVIEWLabVIEWLabVIEWLabVIEWLabVIEWLabVIEWLabVIEWLabVIEWLabVIEWLabVIEWLabVIEWLabVIEWLabVIEWLabVIEWLabVIEWLabVIEWLabVIEWLabVIEWLabVIEWLabVIEWLabVIEWLabVIEWLabVIEWLabVIEWLabVIEWLabVIEWLabVIEWLabVIEWLabVIEWLabVIEWLabVIEWLabVIEWLabVIEWLabVIEWLabVIEWLabVIEWLabVIEWLabVIEWLabVIEWLabVIEWLabVIEWLabVIEWLabVIEWLabVIEWLabVIEWLabVIEWLabVIEWLabVIEWLabVIEWLabVIEWLabVIEWLabVIEWLabVIEWLabVIEWLabVIEWLabVIEWLabVIEWLabVIEWLabVIEWLabVIEWLabVIEWLabVIEWLabVIEWLabVIEWLabVIEWLabVIEWLabVIEWLabVIEWLabVIEWLabVIEWLabVIEWLabVIEWLabVIEWLabVIEWLabVIEWLabVIEWLabVIEWLabVIEWLabVIEWLabVIEWLabVIEWLabVIEWLabVIEWLabVIEWLabVIEWLabVIEWLabVIEWLabVIEWLabVIEWLabVIEWLabVIEWLabVIEWLabVIEWLabVIEWLabVIEWLabVIEWLabVIEWLabVIEWLabVIEWLabVIEWLabVIEWLabVIEWLabVIEWLabVIEWLabVIEWLabVIEWLabVIEWLabVIEWLabVIEWLabVIEWLabVIEWLabVIEWLabVIEWLabVIEWLabVIEWLabVIEWLabVIEWLabVIEWLabVIEWLabVIEWLabVIEWLabVIEWLabVIEWLabVIEWLabVIEWLabVIEWLabVIEWLabVIEWLabVIEWLabVIEWLabVIEWLabVIEWLabVIEWLabVIEWLabVIEWLabVIEWLabVIEWLabVIEWLabVIEWLabVIEWLabVIEWLabVIEWLabVIEWLabVIEWLabVIEWLabVIEWLabVIEWLabVIEWLabVIEWLabVIEWLabVIEWLabVIEWLabVIEWLabVIEWLabVIEWLabVIEWLabVIEWLabVIEWLabVIEWLabVIEWLabVIEWLabVIEWLabVIEWLabVIEWLabVIEWLabVIEWLabVIEWLabVIEWLabVIEWLabVIEWLabVIEWLabVIEWLabVIEWLabVIEWLabVIEWLabVIEWLabVIEWLabVIEWLabVIEWLabVIEWLabVIEWLabVIEWLabVIEWLabVIEWLabVIEWLabVIEWLabVIEWLabVIEWLabVIEWLabVIEWLabVIEWLabVIEWLabVIEWLabVIEWLabVIEWLabVIEWLabVIEWLabVIEWLabVIEWLabVIEWLabVIEWLabVIEWLabVIEWLabVIEWLabVIEWLabVIEWLabVIEWLabVIEWLabVIEWLabVIEWLabVIEWLabVIEWLabVIEWLabVIEWLabVIEWLabVIEWLabVIEWLabVIEWLabVIEWLabVIEWLabVIEWLabVIEWLabVIEWLabVIEWLabVIEWLabVIEWLabVIEWLabVIEWLabVIEWLabVIEWLabVIEWLabVIEWLabVIEWLabVIEWLabVIEWLabVIEWLabVIEWLabVIEWLabVIEWLabVIEWLabVIEWLabVIEWLabVIEWLabVIEWLabVIEWLabVIEWLabVIEWLabVIEWLabVIEWLabVIEWLabVIEWLabVIEWLabVIEWLabVIEWLabVIEWLabVIEWLabVIEWLabVIEWLabVIEWLabVIEWLabVIEWLabVIEWLabVIEWLabVIEWLabVIEWLabVIEWLabVIEWLabVIEWLabVIEWLabVIEWLabVIEWLabVIñ\u0010"], ["QWERTYDSAQWERTYDSAQWERTYDSAQWERTYDSAQWERTYDSAQWERTYDSAQWERTYDSAQWERTYDSAQWERTYDSAQWERTYDSAQWERTYDSAQWERTYDSAQWERTYDSAQWERTYDSAQWERTYDSAQWERTYDSAQWERTYDSAQWERTYDSAQWERTYDSAQWERTYDSAQWERTYDSAQWERTYDSAQWERTYDSAQWERTYDSAQWERTYDSAQWERTYDSAQWERTYDSAQWERTYDSAQWERTYDSAQWERTYDSAQWERTYDSAQWERTYDSAQWERTYDSAQWERTYDSAQWERTYDSAQWERTYDSAQWERTYDSAQWERTYDSAQWERTYDSAQWERTYDSAQWERTYDSAQWERTYDSAQWERTYDSAQWERTYDSAQWERTYDSAQWERTYDSAQWERTYDSAQWERTYDSAQWERTYDSAQWERTYDSAQWERTYDSAQWERTYDSAQWERTYDSAQWERTYDSAQWERTYDSAQWERTYDSAQWERTYDSAQWERTYDSAQWERTYDSAQWERTYDSAQWERTYDSAQWERTYDSAQWERTYDSAQWERTYDSAQWERTYDSAQWERTYDSAQWERTYDSAQWERTYDSAQWERTYDSAQWERTYDSAQWERTYDSAQWERTYDSAQWERTYDSAQWERTYDSAQWERTYDSAQWERTYDSAQWERTYDSAQWERTYDSAQWERTYDSAQWERTYDSAQWERTYDSAQWERTYDSAQWERTYDSAQWERTYDSAQWERTYDSAQWERTYDSAQWERTYDSAQWERTYDSAQWERTYDSAQWERTYDSAQWERTYDSAQWERTYDSAQWERTYDSAQWERTYDSAQWERTYDSAQWERTYDSAQWERTYDSAQWERTYDSAQWERTYDSAQWERTYDSAQWERTYDSAQWERTYDSAQWERTYDSAQWERTYDSAQWERTYDSAQWERTYDSAQWERTYDSAQWERTYDSAQWERTYDSAQWERTYDSAQWERTYDSAQWERTYDSAQWERTYDSAQWERTYDSAQWERTYDSAQWERTYDSAQWERTYDSAQWERTYDSAQWERTYDSAQWERTYDSAQWERTYDSAQWERTYDSAQWERTYDSAQWERTYDSAQWERTYDSAQWERTYDSAQWERTYDSAQWERTYDSAQWERTYDSAQWERTYDSAQWERTYDSAQWERTYDSAQWERTYDSAQWERTYDSAQWERTYDSAQWERTYDSAQWERTYDSAQWERTYDSAQWERTYDSAQWERTYDSAQWERTYDSAQWERTYDSAQWERTYDSAQWERTYDSAQWERTYDSAQWERTYDSAQWERTYDSAQWERTYDSAQWERTYDSAQWERTYDSAQWERTYDSAQWERTYDSAQWERTYDSAQWERTYDSAQWERTYDSAQWERTYDSAQWERTYDSAQWERTYDSAQWERTYDSAQWERTYDSAQWERTYDSAQWERTYDSAQWERTYDSAQWERTYDSAQWERTYDSAQWERTYDSAQWERTYDSAQWERTYDSAQWERTYDSAQWERTYDSAQWERTYDSAQWERTYDSAQWERTYDSAQWERTYDSAQWERTYDSAQWERTYDSAQWERTYDSAQWERTYDSAQWERTYDSAQWERTYDSAQWERTYDSAQWERTYDSAQWERTYDSAQWERTYDSAQWERTYDSAQWERTYDSAQWERTYDSAQWERTYDSAQWERTYDSAQWERTYDSAQWERTYDSAQWERTYDSAQWERTYDSAQWERTYDSAQWERTYDSAQWERTYDSAQWERTYDSAQWERTYDSAQWERTYDSAQWERTYDSAQWERTYDSAQWERTYDSAQWERTYDSAQWERTYDSAQWERTYDSAQWERTYDSAQWERTYDSAQWERTYDSAQWERTYDSAQWERTYDSAQWERTYDSAQWERTYDSAQWERTYDSAQWERTYDSAQWERTYDSAQWERTYDSAQWERTYDSAQWERTYDSAQWERTYDSAQWERTYDSAQWERTYDSAQWERTYDSAQWERTYDSAQWERTYDSAQWERTYDSAQWERTYDSAQWERTYDSAQWERTYDSAQWERTYDSAQWERTYDSAQWERTYDSAQWERTYDSAQWERTYDSAQWERTYDSAQWERTYDSAQWERTYDSAQWERTYDSAQWERTYDSAQWERTYDSAQWERTYDSAQWERTYDSAQWERTYDSAQWERTYDSAQWERTYDSAQWERTYDSAQWERTYDSAQWERTYDSAQWERTYDSAQWERTYDSAQWERTYDSAQWERTYDSAQWERTYDSAQWERTYDSAQWERTYDSAQWERTYDSAQWERTYDSAQWERTYDSAQWERTYDSAQWERTYDSAQWERTYDSAQWERTYDSAQWERTYDSAQWERTYDSAQWERTYDSAQWERTYDSAQWERTYDSAQWERTYDSAQWERTYDSAQWERTYDSAQWERTYDSAQWERTYDSAQWERTYDSAQWERTYDSAQWERTYDSAQWERTYDSAQWERTYDSAQWERTYDSAQWERTYDSAQWERTYDSAQWERTYDSAQWERTYDSAQWERTYDSAQWERTYDSAQWERTYDSAQWERTYDSAQWERTYDSAQWERTYDSAQWERTYDSAQWERTYDSAQWERTYDSAQWERTYDSAQWERTYDSAQWERTYDSAQWERTYDSAQWERTYDSAQWERTYDSAQWERTYDSAQWERTYDSAQWERTYDSAQWERTYDSAQWERTYDSAQWERTYDSAQWERTYDSAQWERTYDSAQWERTYDSAQWERTYDSAQWERTYDSAQWERTYDSAQWERTYDSAQWERTYDSAQWERTYDSAQWERTYDSAQWERTYDSAQWERTYDSAQWERTYDSAQWERTYDSAQWERTYDSAQWERTYDSAQWERTYDSAQWERTYDSAQWERTYDSAQWERTYDSAQWERTYDSAQWERTYDSAQWERTYDSAQWERTYDSAQWERTYDSAQWERTYDSAQWERTYDSAQWERTYDSAQWERTYDSAQWERTYDSAQWERTYDSAQWERTYDSAQWERTYDSAQWERTYDSAQWERTYDSAQWERTYDSAQWERTYDSAQWERTYDSAQWERTYDSAQWERTYDSAQWERTYDSAQWERTYDSAQWERTYDSAQWERTYDSAQWERTYDSAQWERTYDSAQWERTYDSAQWERTYDSAQWERTYDSAQWERTYDSAQWERTYDSAQWERTYDSAQWERTYDSAQWERTYDSAQWERTYDSAQWERTYDSAQWERTYDSAQWERTYDSAQWERTYDSAQWERTYDSAQWERTYDSAQWERTYDSAQWERTYDSAQWERTYDSAQWERTYDSAQWERTYDSAQWERTYDSAQWERTYDSAQWERTYDSAQWERTYDSAQWERTYDSAQWERTYDSAQWERTYDSAQWERTYDSAQWERTYDSAQWERTYDSAQWERTYDSAQWERTYDSAQWERTYDSAQWERTYDSAQWERTYDSAQWERTYDSAQWERTYDSAQWERTYDSAQWERTYDSAQWERTYDSAQWERTYDSAQWERTYDSAQWERTYDSAQWERTYDSAQWERTYDSAQWERTYDSAQWERTYDSAQWERTYDSAQWERTYDSAQWERTYDSAQWERTYDSAQWERTYDSAQWERTYDSAQWERTYDSAQWERTYDSAQWERTYDSAQWERTYDSAQWERTYDSAQWERTYDSAQWERTYDSAQWERTYDSAQWERTYDSAQWERTYDSAQWERTYDSAQWERTYDSAQWERTYDSAQWERTYDSAQWERTYDSAQWERTYDSAQWERTYDSAQWERTYDSAQWERTYDSAQWERTYDSAQWERTYDSAQWERTYDSAQWERTYDSAQWERTYDSAQWERTYDSAQWERTYDSAQWERTYDSAQWERTYDSAQWERTYDSAQWERTYDSAQWERTYDSAQWERTYDSAQWERTYDSAQWERTYDSAQWERTYDSAQWERTYDSAQWERTYDSAQWERTYDSAQWERTYDSAQWERTYDSAQWERTYDSAQWERTYDSAQWERTYDSAQWERTYDSAQWERTYDSAQWERTYDSAQWERTYDSAQWERTYDSAQWERTYDSAQWERTYDSAQWERTYDSAQWERTYDSAQWERTYDSAQWERTYDSAQWERTYDSAQWERTYDSAQWERTYDSAQWERTYDSAQWERTYDSAQWERTYDSAQWERTYDSAQWERTYDSAQWERTYDSAQWERTYDSAQWERTYDSAQWERTYDSAQWERTYDSAQWERTYDSAQWERTYDSAQWERTYDSAQWERTYDSAQWERTYDSAQWERTYDSAQWERTYDSAQWERTYDSAQWERTYDSAQWERTYDSAQWERTYDSAQWERTYDSAQWERTYDSAQWERTYDSAQWERTYDSAQWERTYDSAQWERTYDSAQWERTYDSAQWERTYDSAQWERTYDSAQWERTYDSAQWERTYDSAQWERTYDSAQWERTYDSAQWERTYDSAQWERTYDSAQWERTYDSAQWERTYDSAQWERTYDSAQWERTYDSAQWERTYDSAQWERTYDSAQWERTYDSAQWERTYDSAQWERTYDSAQWERTYDSAQWERTYDSAQWERTYDSAQWERTYDSAQWERTYDSAQWERTYDSAQWERTYDSAQWERTYDSAQWERTYDSAQWERTYDSAQWERTYDSAQWERTYDSAQWERTYDSAQWERTYDSAQWERTYDSAQWERTYDSAQWERTYDSAQWERTYDSAQWERTYDSAQWERTYDSAQWERTYDSAQWERTYDSAQWERTYDSAQWERTYDSAQWERTYDSAQWERTYDSAQWERTYDSAQWERTYDSAQWERTYDSAQWERTYDSAQWERTYDSAQWERTYDSAQWERTYDSAQWERTYDSAQWERTYDSAQWERTYDSAQWERTYDSAQWERTYDSAQWERTYDSAQWERTYDSAQWERTYDSAQWERTYDSAQWERTYDSAQWERTYDSAQWERTYDSAQWERTYDSAQWERTYDSAQWERTYDSAQWERTYDSAQWERTYDSAQWERTYDSAQWERTYDSAQWERTYDSAQWERTYDSAQWERTYDSAQWERTYDSAQWERTYDSAQWERTYDSAQWERTYDSAQWERTYDSAQWERTYDSAQWERTYDSAQWERTYDSAQWERTYDSAQWERTYDSAQWERTYDSAQWERTYDSAQWERTYDSAQWERTYDSAQWERTYDSAQWERTYDSAQWERTYDSAQWERTYDSAQWERTYDSAQWERTYDSAQWERTYDSAQWERTYDSAQWERTYDSAQWERTYDSAQWERTYDSAQWERTYDSAQWERTYDSAQWERTYDSAQWERTYDSAQWERTYDSAQWERTYDSAQWERTYDSAQWERTYDSAQWERTYDSAQWERTYDSAQWERTYDSAQWERTYDSAQWERTYDSAQWERTYDSAQWERTYDSAQWERTYDSAQWERTYDSAQWERTYDSAQWERTYDSAQWERTYDSAQWERTYDSAQWERTYDSAQWERTYDSAQWERTYDSAQWERTYDSAQWERTYDSAQWERTYDSAQWERTYDSAQWERTYDSAQWERTYDSAQWERTYDSAQWERTYDSAQWERTYDSAQWERTYDSAQWERTYDSAQWERTYDSAQWERTYDSAQWERTYDSAQWERTYDSAQWERTYDSAQWERTYDSAQWERTYDSAQWERTYDSAQWERTYDSAQWERTYDSAQWERTYDSAQWERTYDSAQWERTYDSAQWERTYDSAQWERTYDSAQWERTYDSAQWERTYDSAQWERTYDSAQWERTYDSAQWERTYDSAQWERTYDSAQWERTYDSAQWERTYDSAQWERTYDSAQWERTYDSAQWERTYDSAQWERTYDSAQWERTYDSAQWERTYDSAQWERTYDSAQWERTYDSAQWERTYDSAQWERTYDSAQWERTYDSAQWERTYDSAQWERTYDSAQWERTYDSAQWERTYDSAQWERTYDSAQWERTYDSAQWERTYDSAQWERTYDSAQWERTYDSAQWERTYDSAQWERTYDSAQWERTYDSAQWERTYDSAQWERTYDSAQWERTYDSAQWERTYDSAQWERTYDSAQWERTYDSAQWERTYDSAQWERTYDSAQWERTYDSAQWERTYDSAQWERTYDSAQWERTYDSAQWERTYDSAQWERTYDSAQWERTYDSAQWERTYDSAQWERTYDSAQWERTYDSAQWERTYDSAQWERTYDSAQWERTYDSAQWERTYDSAQWERTYDSAQWERTYDSAQWERTYDSAQWERTYDSAQWERTYDSAQWERTYDSAQWERTYDSAQWERTYDSAQWERTYDSAQWERTYDSAQWERTYDSAQWERTYDSAQWERTYDSAQWERTYDSAQWERTYDSAQWERTYDSAQWERTYDSAQWERTYDSAQWERTYDSAQWERTYDSAQWERTYDSAQWERTYDSAQWERTYDSAQWERTYDSAQWERTYDSAQWERTYDSAQWERTYDSAQWERTYDSAQWERTYDSAQWERTYDSAQWERTYDSAQWERTYDSAQWERTYDSAQWERTYDSAQWERTYDSAQWERTYDSAQWERTYDSAQWERTYDSAQWERTYDSAQWERTYDSAQWERTYDSAQWERTYDSAQWERTYDSAQWERTYDSAQWERTYDSAQWERTYDSAQWERTYDSAQWERTYDSAQWERTYDSAQWERTYDSAQWERTYDSAQWERTYDSAQWERTYDSAQWERTYDSAQWERTYDSAQWERTYDSAQWERTYDSAQWERTYDSAQWERTYDSAQWERTYDSAQWERTYDSAQWERTYDSAQWERTYDSAQWERTYDSAQWERTYDSAQWERTYDSAQWERTYDSAQWERTYDSAQWERTYDSAQWERTYDSAQWERTYDSAQWERTYDSAQWERTYDSAQWERTYDSAQWERTYDSAQWERTYDSAQWERTYDSAQWERTYDSAQWERTYDSAQWERTYDSAQWERTYDSAQWERTYDSAQWERTYDSAQWERTYDSAQWERTYDSAQWERTYDSAQWERTYDSAQWERTYDSAQWERTYDSAQWERTYDSAQWERTYDSAQWERTYDSAQWERTYDSAQWERTYDSAQWERTYDSAQWERTYDSAQWERTYDSAQWERTYDSAQWERTYDSAQWERTYDSAQWERTYDSAQWERTYDSAQWERTYDSAQWERTYDSAQWERTYDSAQWERTYDSAQWERTYDSAQWERTYDSAQWERTYDSAQWERTYDSAQWERTYDSAQWERTYDSAQWERTYDSAQWERTYDSAQWERTYDSAQWERTYDSAQWERTYDSAQWERTYDSAQWERTYDSAQWERTYDSAQWERTYDSAQWERTYDSAQWERTYDSAQWERTYDSAQWERTYDSAQWERTYDSAQWERTYDSAQWERTYDSAQWERTYDSAQWERTYDSAQWERTYDSAQWERTYDSAQWERTYDSAQWERTYDSAQWERTYDSAQWERTYDSAQWERTYDSAQWERTYDSAQWERTYDSAQWERTYDSAQWERTYDSAQWERTYDSAQWERTYDSAQWERTYDSAQWERTYDSAQWERTYDSAQWERTYDSAQWERTYDSAQWERTYDSAQWERTYDSAQWERTYDSAQWERTYDSAQWERTYDSAQWERTYDSAQWERTYDSAQWERTYDSAQWERTYDSAQWERTYDSAQWERTYDSAQWERTYDSAQWERTYDSAQWERTYDSAQWERTYDSAQWERTYDSAQWERTYDSAQWERTYDSAQWERTYDSAQWERTYDSAQWERTYDSAQWERTYDSAQWERTYDSAQWERTYDSAQWERTYDSAQWERTYDSAQWERTYDSAQWERTYDSAQWERTYDSAQWERTYDSAQWERTYDSAQWERTYDSAQWERTYDSAQWERTYDSAQWERTYDSAQWERTYDSAQWERTYDSAQWERTYDSAQWERTYDSAQWERTYDSAQWERTYDSAQWERTYDSAQWERTYDSAQWERTYDSAQWERTYDSAQWERTYDSAQWERTYDSAQWERTYDSAQWERTYDSAQWERTYDSAQWERTYDSAQWERTYDSAQWERTYDSAQWERTYDSAQWERTYDSAQWERTYDSAQWERTYDSAQWERTYDSAQWERTYDSAQWERTYDSAQWERTYDSAQWERTYDSAQWERTYDSAQWERTYDSAQWERTYDSAQWERTYDSAQWERTYDSAQWERTYDSAQWERTYDSAQWERTYDSAQWERTYDSAQWERTYDSAQWERTYDSAQWERTYDSAQWERTYDSAQWERTYDSAQWERTYDSAQWERTYDSAQWERTYDSAQWERTYDSAQWERTYDSAQWERTYDSAQWERTYDSAQWERTYDSAQWERTYDSAQWERTYDSAQWERTYDSAQWERTYDSAQWERTYDSAQWERTYDSAQWERTYDSAQWERTYDSAQWERTYDSAQWERTYDSAQWERTYDSAQWERTYDSAQWERTYDSAQWERTYDSAQWERTYDSAQWERTYDSAQWERTYDSAQWERTYDSAQWERTYDSAQWERTYDSAQWERTYDSAQWERTYDSAQWERTYDSAQWERTYDSAQWERTYDSAQWERTYDSAQWERTYDSAQWERTYDSAQWERTYDSAQWERTYDSAQWERTYDSAQWERTYDSAQWERTYDSAQWERTYDSAQWERTYDSAQWERTYDSAQWERTYDSAQWERTYDSAQWERTYDSAQWERTYDSAQWERTYDSAQWERTYDSAQWERTYDSAQWERTYDSAQWERTYDSAQWERTYDSAQWERTYDSAQWERTYDSAQWERTYDSAQWERTYDSAQWERTYDSAQWERTYDSAQWERTYDSAQWERTYDSAQWERTYDSAQWERTYDSAQWERTYDSAQWERTYDSAQWERTYDSAQWERTYDSAQWERTYDSAQWERTYDSAQWERTYDSAQWERTYDSAQWERTYDSAQWERTYDSAQWERTYDSAQWERTYDSAQWERTYDSAQWERTYDSAQWERTYDSAQWERTYDSAQWERTYDSAQWERTYDSAQWERTYDSAQWERTYDSAQWERTYDSAQWERTYDSAQWERTYDSAQWERTYDSAQWERTYDSAQWERTYDSA͠", "~~w~~w~~w~~w~~w~~w~~w~~w~~w~~w~~w~~w~~w~~w~~w~~w~~w~~w~~w~~w~~w~~w~~w~~w~~w~~w~~w~~w~~w~~w~~w~~w~~w~~w~~w~~w~~w~~w~~w~~w~~w~~w~~w~~w~~w~~w~~w~~w~~w~~w~~w~~w~~w~~w~~w~~w~~w~~w~~w~~w~~w~~w~~w~~w~~w~~w~~w~~w~~w~~w~~w~~w~~w~~w~~w~~w~~w~~w~~w~~w~~w~~w~~w~~w~~w~~w~~w~~w~~w~~w~~w~~w~~w~~w~~w~~w~~w~~w~~w~~w~~w~~w~~w~~w~~w~~w~~w~~w~~w~~w~~w~~w~~w~~w~~w~~w~~w~~w~~w~~w~~w~~w~~w~~w~~w~~w~~w~~w~~w~~w~~w~~w~~w~~w~~w~~w~~w~~w~~w~~w~~w~~w~~w~~w~~w~~w~~w~~w~~w~~w~~w~~w~~w~~w~~w~~w~~w~~w~~w~~w~~w~~w~~w~~w~~w~~w~~w~~w~~w~~w~~w~~w~~w~~w~~w~~w~~w~~w~~w~~w~~w~~w~~w~~w~~w~~w~~w~~w~~w~~w~~w~~w~~w~~w~~w~~w~~w~~w~~w~~w~~w~~w~~w~~w~~w~~w~~w~~w~~w~~w~~w~~w~~w~~w~~w~~w~~w~~w~~w~~w~~w~~w~~w~~w~~w~~w~~w~~w~~w~~w~~w~~w~~w~~w~~w~~w~~w~~w~~w~~w~~w~~w~~w~~w~~w~~w~~w~~w~~w~~w~~w~~w~~w~~w~~w~~w~~w~~w~~w~~w~~w~~w~~w~~w~~w~~w~~w~~w~~w~~w~~w~~w~~w~~w~~w~~w~~w~~w~~w~~w~~w~~w~~w~~w~~w~~w~~w~~w~~w~~w~~w~~w~~w~~w~~w~~w~~w~~w~~w~~w~~w~~w~~w~~w~~w~~w~~w~~w~~w~~w~~w~~w~~w~~w~~w~~w~~w~~w~~w~~w~~w~~w~~w~~w~~w~~w~~w~~w~~w~~w~~w~~w~~w~~w~~w~~w~~w~~w~~w~~w~~w~~w~~w~~w~~w~~w~~w~~w~~w~~w~~w~~w~~w~~w~~w~~w~~w~~w~~w~~w~~w~~w~~w~~w~~w~~w~~w~~w~~w~~w~~w~~w~~w~~w~~w~~w~~w~~w~~w~~w~~w~~w~~w~~w~~w~~w~~w~~w~~w~~w~~w~~w~~w~~w~~w~~w~~w~~w~~w~~w~~w~~w~~w~~w~~w~~w~~w~~w~~w~~w~~w~~w~~w~~w~~w~~w~~w~~w~~w~~w~~w~~w~~w~~w~~w~~w~~w~~w~~w~~w~~w~~w~~w~~w~~w~~w~~w~~w~~w~~w~~w~~w~~w~~w~~w~~w~~w~~w~~w~~w~~w~~w~~w~~w~~w~~w~~w~~w~~w~~w~~w~~w~~w~~w~~w~~w~~w~~w~~w~~w~~w~~w~~w~~w~~w~~w~~w~~w~~w~~w~~w~~w~~w~~w~~w~~w~~w~~w~~w~~w~~w~~w~~w~~w~~w~~w~~w~~w~~w~~w~~w~~w~~w~~w~~w~~w~~w~~w~~w~~w~~w~~w~~w~~w~~w~~w~~w~~w~~w~~w~~w~~w~~w~~w~~w~~w~~w~~w~~w~~w~~w~~w~~w~~w~~w~~w~~w~~w~~w~~w~~w~~w~~w~~w~~w~~w~~w~~w~~w~~w~~w~~w~~w~~w~~w~~w~~w~~w~~w~~w~~w~~w~~w~~w~~w~~w~~w~~w~~w~~w~~w~~w~~w~~w~~w~~w~~w~~w~~w~~w~~w~~w~~w~~w~~w~~w~~w~~w~~w~~w~~w~~w~~w~~w~~w~~w~~w~~w~~w~~w~~w~~w~~w~~w~~w~~w~~w~~w~~w~~w~~w~~w~~w~~w~~w~~w~~w~~w~~w~~w~~w~~w~~w~~w~~w~~w~~w~~w~~w~~w~~w~~w~~w~~w~~w~~w~~w~~w~~w~~w~~w~~w~~w~~w~~w~~w~~w~~w~~w~~w~~w~~w~~w~~w~~w~~w~~w~~w~~w~~w~~w~~w~~w~~w~~w~~w~~w~~w~~w~~w~~w~~w~~w~~w~~w~~w~~w~~w~~w~~w~~w~~w~~w~~w~~w~~w~~w~~w~~w~~w~~w~~w~~w~~w~~w~~w~~w~~w~~w~~w~~w~~w~~w~~w~~w~~w~~w~~w~~w~~w~~w~~w~~w~~w~~w~~w~~w~~w~~w~~w~~w~~w~~w~~w~~w~~w~~w~~w~~w~~w~~w~~w~~w~~w~~w~~w~~w~~w~~w~~w~~w~~w~~w~~w~~w~~w~~w~~w~~w~~w~~w~~w~~w~~w~~w~~w~~w~~w~~w~~w~~w~~w~~w~~w~~w~~w~~w~~w~~w~~w~~w~~w~~w~~w~~w~~w~~w~~w~~w~~w~~w~~w~~w~~w~~w~~w~~w~~w~~w~~w~~w~~w~~w~~w~~w~~w~~w~~w~~w~~w~~w~~w~~w~~w~~w~~w~~w~~w~~w~~w~~w~~w~~w~~w~~w~~w~~w~~w~~w~~w~~w~~w~~w~~w~~w~~w~~w~~w~~w~~w~~w~~w~~w~~w~~w~~w~~w~~w~~w~~w~~w~~w~~w~~w~~w~~w~~w~~w~~w~~w~~w~~w~~w~~w~~w~~w~~w~~w~~w~~w~~w~~w~~w~~w~~w~~w~~w~~w~~w~~w~~w~~w~~w~~w~~w~~w~~w~~w~~w~~w~~w~~w~~w~~w~~w~~w~~w~~w~~w~~w~~w~~w~~w~~w~~w~~w~~w~~w~~w~~w~~w~~w~~w~~w~~w~~w~~w~~w~~w~~w~~w~~w~~w~~w~~w~~w~~w~~w~~w~~w~~w~~w~~w~~w~~w~~w~~w~~w~~w~~w~~w~~w~~w~~w~~w~~w~~w~~w~~w~~w~~w~~w~~w~~w~~w~~w~~w~~w~~w~~w~~w~~w~~w~~w~~w~~w~~w~~w~~w~~w~~w~~w~~w~~w~~w~~w~~w~~w~~w~~w~~w~~w~~w~~w~~w~~w~~w~~w~~w~~w~~w~~w~~w~~w~~w~~w~~w~~w~~w~~w~~w~~w~~w~~w~~w~~w~~w~~w~~w~~w©8", "abcdabcdabcdabcdabcdabcdabcdabcdabcdabcdabcdabcdabcdabcdabcdabcdabcdabcdabcdabcdabcdabcdabcdabcdabcdabcdabcdabcdabcdabcdabcdabcdabcdabcdabcdabcdabcdabcdabcdabcdabcdabcdabcdabcdabcdabcdabcdabcdabcdabcdabcdabcdabcdabcdabcdabcdabcdabcdabcdabcdabcdabcdabcdabcdabcdabcdabcdabcdabcdabcdabcdabcdabcdabcdabcdabcdabcdabcdabcdabcdabcdabcdabcdabcdabcdabcdabcdabcdabcdabcdabcdabcdabcdabcdabcdabcdabcdabcdabcdabcdabcdabcdabcdabcdabcdabcdabcdabcdabcdabcdabcdabcdabcdabcdabcdabcdabcdabcdabcdabcdabcdabcdabcdabcdabcdabcdabcdabcdabcdabcdabcdabcdabcdabcdabcdabcdabcdabcdabcdabcdabcdabcdabcdabcdabcdabcdabcdabcdabcdabcdabcdabcdabcdabcdabcdabcdabcdabcdabcdabcdabcdabcdabcdabcdabcdabcdabcdabcdabcdabcdabcdabcdabcdabcdabcdabcdabcdabcdabcdabcdabcdabcdabcdabcdabcdabcdabcdabcdabcdabcdabcdabcdabcdabcdabcdabcdabcdabcdabcdabcdabcdabcdabcdabcdabcdabcdabcdabcdabcdabcdabcdabcdabcdabcdabcdabcdabcdabcdabcdabcdabcdabcdabcdabcdabcdabcdabcdabcdabcdabcdabcdabcdabcdabcdabcdabcdabcdabcdabcdabcdabcdabcdabcdabcdabcdabcdabcdabcdabcdabcdabcdabcdabcdabcdabcdabcdabcdabcdabcdabcdabcdabcdabcdabcdabcdabcdabcdabcdabcdabcdabcdabcdabcdabcdabcdabcdabcdabcdabcdabcdabcdabcdabcdabcdabcdabcdabcdabcdabcdabcdabcdabcdabcdabcdabcdabcdabcdabcdabcdabcdabcdabcdabcdabcdabcdabcdabcdabcdabcdabcdabcdabcdabcdabcdabcdabcdabcdabcdabcdabcdabcdabcdabcdabcdabcdabcdabcdabcdabcdabcdabcdabcdabcdabcdabcdabcdabcdabcdabcdabcdabcdabcdabcdabcdabcdabcdabcdabcdabcdabcdabcdabcdabcdabcdabcdabcdabcdabcdabcdabcdabcdabcdabcdabcdabcdabcdabcdabcdabcdabcdabcdabcdabcdabcdabcdabcdabcdabcdabcdabcdabcdabcdabcdabcdabcdabcdabcdabcdabcdabcdabcdabcdabcdabcdabcdabcdabcdabcdabcdabcdabcdabcdabcdabcdabcdabcdabcdabcdabcdabcdabcdabcdabcdabcdabcdabcdabcdabcdabcdabcdabcdabcdabcdabcdabcdabcdabcdabcdabcdabcdabcdabcdabcdabcdabcdabcdabcdabcdabcdabcdabcdabcdabcdabcdabcdabcdabcdabcdabcdabcdabcdabcdabcdabcdabcdabcdabcdabcdabcdabcdabcdabcdabcdabcdabcdabcdabcdabcdabcdabcdabcdabcdabcdabcdabcdabcdabcdabcdabcdabcdabcdabcdabcdabcdabcdabcdabcdabcdabcdabcdabcdabcdabcdabcdabcdabcdabcdabcdabcdabcdabcdabcdabcdabcdabcdabcdabcdabcdabcdabcdabcdabcdabcdabcdabcdabcdabcdabcdabcdabcdabcdabcdabcdabcdabcdabcdabcdabcdabcdabcdabcdabcdabcdabcdabcdabcdabcdabcdabcdabcdabcdabcdabcdabcdabcdabcdabcdabcdabcdabcdabcdabcdabcdabcdabcdabcdabcdabcdabcdabcdabcdabcdabcdabcdabcdabcdabcdabcdabcdabcdabcdabcdabcdabcdabcdabcdabcdabcdabcdabcdabcdabcdabcdabcdabcdabcdabcdabcdabcdabcdabcdabcdabcdabcdabcdabcdabcdabcdabcdabcdabcdabcdabcdabcdabcdabcdabcdabcdabcdabcdabcdabcdabcdabcdabcdabcdabcdabcdabcdabcdabcdabcdabcdabcdabcdabcdabcdabcdabcdabcdabcdabcdabcdabcdabcdabcdabcdabcdabcdabcdabcdabcdabcdabcdabcdabcdabcdabcdabcdabcdabcdabcdabcdabcdabcdabcdabcdabcdabcdabcdabcdabcdabcdabcdabcdabcdabcdabcdabcdabcdabcdabcdabcdabcdabcdabcdabcdabcdabcdabcdabcdabcdabcdabcdabcdabcdabcdabcdabcdabcdabcdabcdabcdabcdabcdabcdabcdabcdabcdabcdabcdabcdabcdabcdabcdabcdabcdabcdabcdabcdabcdabcdabcdabcdabcdabcdabcdabcdabcdabcdabcdabcdabcdabcdabcdabcdabcdabcdabcdabcdabcdabcdabcdabcdabcdabcdabcdabcdabcdabcdabcdabcdabcdabcdabcdabcdabcdabcdabcdabcdabcdabcdabcdabcdabcdabcdabcdabcdabcdabcdabcdabcdabcdabcdabcdabcdabcdabcdabcdabcdabcdabcdabcdabcdabcdabcdabcdabcdabcdabcdabcdabcdabcdabcdabcdabcdabcdabcdabcdabcdabcdabcdabcdabcdabcdabcdabcdabcdabcdabcdabcdabcdabcdabcdabcdabcdabcdabcdabcdabcdabcdabcdabcdabcdabcdabcdabcdabcdabcdabcdabcdabcdabcdabcdabcdabcdabcdabcdabcdabcdabcdabcdabcdabcdabcdabcdabcdabcdabcdabcdabcdabcdabcdabcdabcdabcdabcdabcdabcdabcdabcdabcdabcdabcdabcdabcdabcdabcdabcdabcdabcdabcdabcdabcdabcdabcdabcdabcdabcdabcdabcdabcdabcdabcdabcdabcdabcdabcdabcdabcdabcdabcdabcdabcdabcdabcdabcdabcdabcdabcdabcdabcdabcdabcdabcdabcdabcdabcdabcdabcdabcdabcdabcdabcdabcdabcdabcdabcdabcdabcdabcdabcdabcdabcdabcdabcdabcdabcdabcdabcdabcdabcdabcdabcdabcdabcdabcdabcdabcdabcdabcdabcdabcdabcdabcdabcdabcdabcdabcdabcdabcdabcdabcdabcdabcdabcdabcdabcdabcdabcdabcdabcdabcdabcdabcdabcdabcdabcdabcdabcdabcdabcdabcdabcdabcdabcdabcdabcdabcdabcdabcdabcdabcdabcdabcdabcdabcdabcdabcdabcdabcdabcdabcdabcdabcdabcdabcdabcdabcdabcdabcdabcdabcdabcdabcdabcdabcdabcdabcdabcd\u0003\u0010", "__dsa/.432__dsa/.432__dsa/.432__dsa/.432__dsa/.432__dsa/.432__dsa/.432__dsa/.432__dsa/.432__dsa/.432__dsa/.432__dsa/.432__dsa/.432__dsa/.432__dsa/.432__dsa/.432__dsa/.432__dsa/.432__dsa/.432__dsa/.432__dsa/.432__dsa/.432__dsa/.432__dsa/.432__dsa/.432__dsa/.432__dsa/.432__dsa/.432__dsa/.432__dsa/.432__dsa/.432__dsa/.432__dsa/.432__dsa/.432__dsa/.432__dsa/.432__dsa/.432__dsa/.432__dsa/.432__dsa/.432__dsa/.432__dsa/.432__dsa/.432__dsa/.432__dsa/.432__dsa/.432__dsa/.432__dsa/.432__dsa/.432__dsa/.432__dsa/.432__dsa/.432__dsa/.432__dsa/.432__dsa/.432__dsa/.432__dsa/.432__dsa/.432__dsa/.432__dsa/.432__dsa/.432__dsa/.432__dsa/.432__dsa/.432__dsa/.432__dsa/.432__dsa/.432__dsa/.432__dsa/.432__dsa/.432__dsa/.432__dsa/.432__dsa/.432__dsa/.432__dsa/.432__dsa/.432__dsa/.432__dsa/.432__dsa/.432__dsa/.432__dsa/.432__dsa/.432__dsa/.432__dsa/.432__dsa/.432__dsa/.432__dsa/.432__dsa/.432__dsa/.432__dsa/.432__dsa/.432__dsa/.432__dsa/.432__dsa/.432__dsa/.432__dsa/.432__dsa/.432__dsa/.432__dsa/.432__dsa/.432__dsa/.432__dsa/.432__dsa/.432__dsa/.432__dsa/.432__dsa/.432__dsa/.432__dsa/.432__dsa/.432__dsa/.432__dsa/.432__dsa/.432__dsa/.432__dsa/.432__dsa/.432__dsa/.432__dsa/.432__dsa/.432__dsa/.432__dsa/.432__dsa/.432__dsa/.432__dsa/.432__dsa/.432__dsa/.432__dsa/.432__dsa/.432__dsa/.432__dsa/.432__dsa/.432__dsa/.432__dsa/.432__dsa/.432__dsa/.432__dsa/.432__dsa/.432__dsa/.432__dsa/.432__dsa/.432__dsa/.432__dsa/.432__dsa/.432__dsa/.432__dsa/.432__dsa/.432__dsa/.432__dsa/.432__dsa/.432__dsa/.432__dsa/.432__dsa/.432__dsa/.432__dsa/.432__dsa/.432__dsa/.432__dsa/.432__dsa/.432__dsa/.432__dsa/.432__dsa/.432__dsa/.432__dsa/.432__dsa/.432__dsa/.432__dsa/.432__dsa/.432__dsa/.432__dsa/.432__dsa/.432__dsa/.432__dsa/.432__dsa/.432__dsa/.432__dsa/.432__dsa/.432__dsa/.432__dsa/.432__dsa/.432__dsa/.432__dsa/.432__dsa/.432__dsa/.432__dsa/.432__dsa/.432__dsa/.432__dsa/.432__dsa/.432__dsa/.432__dsa/.432__dsa/.432__dsa/.432__dsa/.432__dsa/.432__dsa/.432__dsa/.432__dsa/.432__dsa/.432__dsa/.432__dsa/.432__dsa/.432__dsa/.432__dsa/.432__dsa/.432__dsa/.432__dsa/.432__dsa/.432__dsa/.432__dsa/.432__dsa/.432__dsa/.432__dsa/.432__dsa/.432__dsa/.432__dsa/.432__dsa/.432__dsa/.432__dsa/.432__dsa/.432__dsa/.432__dsa/.432__dsa/.432__dsa/.432__dsa/.432__dsa/.432__dsa/.432__dsa/.432__dsa/.432__dsa/.432__dsa/.432__dsa/.432__dsa/.432__dsa/.432__dsa/.432__dsa/.432__dsa/.432__dsa/.432__dsa/.432__dsa/.432__dsa/.432__dsa/.432__dsa/.432__dsa/.432__dsa/.432__dsa/.432__dsa/.432__dsa/.432__dsa/.432__dsa/.432__dsa/.432__dsa/.432__dsa/.432__dsa/.432__dsa/.432__dsa/.432__dsa/.432__dsa/.432__dsa/.432__dsa/.432__dsa/.432__dsa/.432__dsa/.432__dsa/.432__dsa/.432__dsa/.432__dsa/.432__dsa/.432__dsa/.432__dsa/.432__dsa/.432__dsa/.432__dsa/.432__dsa/.432__dsa/.432__dsa/.432__dsa/.432__dsa/.432__dsa/.432__dsa/.432__dsa/.432__dsa/.432__dsa/.432__dsa/.432__dsa/.432__dsa/.432__dsa/.432__dsa/.432__dsa/.432__dsa/.432__dsa/.432__dsa/.432__dsa/.432__dsa/.432__dsa/.432__dsa/.432__dsa/.432__dsa/.432__dsa/.432__dsa/.432__dsa/.432__dsa/.432__dsa/.432__dsa/.432__dsa/.432__dsa/.432__dsa/.432__dsa/.432__dsa/.432__dsa/.432__dsa/.432__dsa/.432__dsa/.432__dsa/.432__dsa/.432__dsa/.432__dsa/.432__dsa/.432__dsa/.432__dsa/.432__dsa/.432__dsa/.432__dsa/.432__dsa/.432__dsa/.432__dsa/.432__dsa/.432__dsa/.432__dsa/.432__dsa/.432__dsa/.432__dsa/.432__dsa/.432__dsa/.432__dsa/.432__dsa/.432__dsa/.432__dsa/.432__dsa/.432__dsa/.432__dsa/.432__dsa/.432__dsa/.432__dsa/.432__dsa/.432__dsa/.432__dsa/.432__dsa/.432__dsa/.432__dsa/.432__dsa/.432__dsa/.432__dsa/.432__dsa/.432__dsa/.432__dsa/.432__dsa/.432__dsa/.432__dsa/.432__dsa/.432__dsa/.432__dsa/.432__dsa/.432__dsa/.432__dsa/.432__dsa/.432__dsa/.432__dsa/.432__dsa/.432__dsa/.432__dsa/.432__dsa/.432__dsa/.432__dsa/.432__dsa/.432__dsa/.432__dsa/.432__dsa/.432__dsa/.432__dsa/.432__dsa/.432__dsa/.432__dsa/.432__dsa/.432__dsa/.432__dsa/.432__dsa/.432__dsa/.432__dsa/.432__dsa/.432__dsa/.432__dsa/.432__dsa/.432__dsa/.432__dsa/.432__dsa/.432__dsa/.432__dsa/.432__dsa/.432__dsa/.432__dsa/.432__dsa/.432__dsa/.432__dsa/.432__dsa/.432__dsa/.432__dsa/.432__dsa/.432__dsa/.432__dsa/.432__dsa/.432__dsa/.432__dsa/.432__dsa/.432__dsa/.432__dsa/.432__dsa/.432__dsa/.432__dsa/.432__dsa/.432__dsa/.432__dsa/.432__dsa/.432__dsa/.432__dsa/.432__dsa/.432__dsa/.432__dsa/.432__dsa/.432__dsa/.432__dsa/.432__dsa/.432__dsa/.432__dsa/.432__dsa/.432__dsa/.432__dsa/.432__dsa/.432__dsa/.432__dsa/.432__dsa/.432__dsa/.432__dsa/.432__dsa/.432__dsa/.432__dsa/.432__dsa/.432__dsa/.432__dsa/.432__dsa/.432__dsa/.432__dsa/.432__dsa/.432__dsa/.432__dsa/.432__dsa/.432__dsa/.432__dsa/.432__dsa/.432__dsa/.432__dsa/.432__dsa/.432__dsa/.432__dsa/.432__dsa/.432__dsa/.432__dsa/.432__dsa/.432__dsa/.432__dsa/.432__dsa/.432__dsa/.432__dsa/.432__dsa/.432__dsa/.432__dsa/.432__dsa/.432__dsa/.432__dsa/.432__dsa/.432__dsa/.432__dsa/.432__dsa/.432__dsa/.432__dsa/.432__dsa/.432__dsa/.432__dsa/.432__dsa/.432__dsa/.432__dsa/.432__dsa/.432__dsa/.432__dsa/.432__dsa/.432__dsa/.432__dsa/.432__dsa/.432__dsa/.432__dsa/.432__dsa/.432__dsa/.432__dsa/.432__dsa/.432__dsa/.432__dsa/.432__dsa/.432__dsa/.432__dsa/.432__dsa/.432__dsa/.432__dsa/.432__dsa/.432__dsa/.432__dsa/.432__dsa/.432__dsa/.432__dsa/.432__dsa/.432__dsa/.432__dsa/.432__dsa/.432__dsa/.432__dsa/.432__dsa/.432__dsa/.432__dsa/.432__dsa/.432__dsa/.432__dsa/.432__dsa/.432__dsa/.432__dsa/.432__dsa/.432__dsa/.432__dsa/.432__dsa/.432__dsa/.432__dsa/.432__dsa/.432__dsa/.432__dsa/.432__dsa/.432__dsa/.432__dsa/.432__dsa/.432__dsa/.432__dsa/.432__dsa/.432__dsa/.432__dsa/.432__dsa/.432__dsa/.432__dsa/.432__dsa/.432__dsa/.432__dsa/.432__dsa/.432__dsa/.432__dsa/.432__dsa/.432__dsa/.432__dsa/.432__dsa/.432__dsa/.432__dsa/.432__dsa/.432__dsa/.432__dsa/.432__dsa/.432__dsa/.432__dsa/.432__dsa/.432__dsa/.432__dsa/.432__dsa/.432__dsa/.432__dsa/.432__dsa/.432__dsa/.432__dsa/.432__dsa/.432__dsa/.432__dsa/.432__dsa/.432__dsa/.432__dsa/.432__dsa/.432__dsa/.432__dsa/.432__dsa/.432__dsa/.432__dsa/.432__dsa/.432__dsa/.432__dsa/.432__dsa/.432__dsa/.432__dsa/.432__dsa/.432__dsa/.432__dsa/.432__dsa/.432__dsa/.432__dsa/.432__dsa/.432__dsa/.432__dsa/.432__dsa/.432__dsa/.432__dsa/.432__dsa/.432__dsa/.432__dsa/.432__dsa/.432__dsa/.432__dsa/.432__dsa/.432__dsa/.432__dsa/.432__dsa/.432__dsa/.432__dsa/.432__dsa/.432__dsa/.432__dsa/.432__dsa/.432__dsa/.432__dsa/.432__dsa/.432__dsa/.432__dsa/.432__dsa/.432__dsa/.432__dsa/.432__dsa/.432__dsa/.432__dsa/.432__dsa/.432__dsa/.432__dsa/.432__dsa/.432__dsa/.432__dsa/.432__dsa/.432__dsa/.432__dsa/.432__dsa/.432__dsa/.432__dsa/.432__dsa/.432__dsa/.432__dsa/.432__dsa/.432__dsa/.432__dsa/.432__dsa/.432__dsa/.432__dsa/.432__dsa/.432__dsa/.432__dsa/.432__dsa/.432__dsa/.432__dsa/.432__dsa/.432__dsa/.432__dsa/.432__dsa/.432__dsa/.432__dsa/.432__dsa/.432__dsa/.432__dsa/.432__dsa/.432__dsa/.432__dsa/.432__dsa/.432__dsa/.432__dsa/.432__dsa/.432__dsa/.432__dsa/.432__dsa/.432__dsa/.432__dsa/.432__dsa/.432__dsa/.432__dsa/.432__dsa/.432__dsa/.432__dsa/.432__dsa/.432__dsa/.432__dsa/.432__dsa/.432__dsa/.432__dsa/.432__dsa/.432__dsa/.432__dsa/.432__dsa/.432__dsa/.432__dsa/.432__dsa/.432__dsa/.432__dsa/.432__dsa/.432__dsa/.432__dsa/.432__dsa/.432__dsa/.432__dsa/.432__dsa/.432__dsa/.432__dsa/.432__dsa/.432__dsa/.432__dsa/.432__dsa/.432__dsa/.432__dsa/.432__dsa/.432__dsa/.432__dsa/.432__dsa/.432__dsa/.432__dsa/.432__dsa/.432__dsa/.432__dsa/.432__dsa/.432__dsa/.432__dsa/.432__dsa/.432__dsa/.432__dsa/.432__dsa/.432__dsa/.432__dsa/.432__dsa/.432__dsa/.432__dsa/.432__dsa/.432__dsa/.432__dsa/.432__dsa/.432__dsa/.432__dsa/.432__dsa/.432__dsa/.432__dsa/.432__dsa/.432__dsa/.432__dsa/.432__dsa/.432__dsa/.432__dsa/.432__dsa/.432__dsa/.432__dsa/.432__dsa/.432__dsa/.432__dsa/.432__dsa/.432__dsa/.432__dsa/.432__dsa/.432__dsa/.432__dsa/.432__dsa/.432__dsa/.432__dsa/.432__dsa/.432__dsa/.432__dsa/.432__dsa/.432__dsa/.432__dsa/.432__dsa/.432__dsa/.432__dsa/.432__dsa/.432__dsa/.432__dsa/.432__dsa/.432__dsa/.432__dsa/.432__dsa/.432__dsa/.432__dsa/.432__dsa/.432__dsa/.432__dsa/.432__dsa/.432__dsa/.432__dsa/.432__dsa/.432__dsa/.432__dsa/.432__dsa/.432__dsa/.432__dsa/.432__dsa/.432__dsa/.432__dsa/.432__dsa/.432__dsa/.432__dsa/.432__dsa/.432__dsa/.432__dsa/.432__dsa/.432__dsa/.432__dsa/.432__dsa/.432__dsa/.432__dsa/.432__dsa/.432__dsa/.432__dsa/.432__dsa/.432__dsa/.432__dsa/.432__dsa/.432__dsa/.432__dsa/.432__dsa/.432__dsa/.432__dsa/.432__dsa/.432__dsa/.432__dsa/.432__dsa/.432__dsa/.432__dsa/.432__dsa/.432__dsa/.432__dsa/.432__dsa/.432__dsa/.432__dsa/.432__dsa/.432__dsa/.432__dsa/.432__dsa/.432__dsa/.432__dsa/.432__dsa/.432__dsa/.432__dsa/.432__dsa/.432__dsa/.432__dsa/.432__dsa/.432__dsa/.432__dsa/.432__dsa/.432__dsa/.432__dsa/.432__dsa/.432__dsa/.432__dsa/.432__dsa/.432__dsa/.432__dsa/.432__dsa/.432__dsa/.432__dsa/.432__dsa/.432__dsa/.432__dsa/.432__dsa/.432__dsa/.432__dsa/.432__dsa/.432__dsa/.432__dsa/.432__dsa/.432__dsa/.432__dsa/.432__dsa/.432__dsa/.432__dsa/.432__dsa/.432__dsa/.432__dsa/.432__dsa/.432__dsa/.432__dsa/.432__dsa/.432__dsa/.432__dsa/.432__dsa/.432__dsa/.432__dsa/.432__dsa/.432__dsa/.432__dsa/.432__dsa/.432__dsa/.432__dsa/.432__dsa/.432__dsa/.432__dsa/.432__dsa/.432__dsa/.432__dsa/.432__dsa/.432__dsa/.432__dsa/.432__dsa/.432__dsa/.432__dsa/.432__dsa/.432__dsa/.432__dsa/.432__dsa/.432__dsa/.432__dsa/.432__dsa/.432__dsa/.432__dsa/.432__dsa/.432__dsa/.432__dsa/.432__dsa/.432__dsa/.432__dsa/.432__dsa/.432__dsa/.432__dsa/.432__dsa/.432__dsa/.432__dsa/.432__dsa/.432__dsa/.432__dsa/.432__dsa/.432__dsa/.432__dsa/.432__dsa/.432__dsa/.432__dsa/.432__dsa/.432__dsa/.432__dsa/.432__dsa/.432__dsa/.432__dsa/.432__dsa/.432__dsa/.432__dsa/.432__dsa/.432__dsa/.432__dsa/.432__dsa/.432__dsa/.432__dsa/.432__dsa/.432__dsa/.432__dsa/.432__dsa/.432__dsa/.432__dsa/.432__dsa/.432__dsa/.432__dsa/.432__dsa/.432__dsa/.432__dsa/.432__dsa/.432__dsa/.432__dsa/.432__dsa/.432__dsa/.432__dsa/.432__dsa/.432__dsa/.432__dsa/.432__dsa/.432__dsa/.432__dsa/.432__dsa/.432__dsa/.432__dsa/.432__dsa/.432__dsa/.432__dsa/.432__dsa/.432__dsa/.432__dsa/.432__dsa/.432__dsa/.432__dsa/.432__dsa/.432__dsa/.432__dsa/.432__dsa/.432__dsa/.432__dsa/.432__dsa/.432ià", "$#$#$#$#$#$#$#$#$#$#$#$#$#$#$#$#$#$#$#$#$#$#$#$#$#$#$#$#$#$#$#$#$#$#$#$#$#$#$#$#$#$#$#$#$#$#$#$#$#$#$#$#$#$#$#$#$#$#$#$#$#$#$#$#$#$#$#$#$#$#$#$#$#$#$#$#$#$#$#$#$#$#$#$#$#$#$#$#$#$#$#$#$#$#$#$#$#$#$#$#$#$#$#$#$#$#$#$#$#$#$#$#$#$#$#$#$#$#$#$#$#$#$#$#$#$#$#$#$#$#$#$#$#$#$#$#$#$#$#$#$#$#$#$#$#$#$#$#$#$#$#$#$#$#$#$#$#$#$#$#$#$#$#$#$#$#$#$#$#$#$#$#$#$#$#$#$#$#$#$#$#$#$#$#$#$#$#$#$#$#$#$#$#$#$#$#$#$#$#$#$#$#$#$#$#$#$#$#$#$#$#$#$#$#$#$#$#$#$#$#$#$#$#$#$#$#$#$#$#$#$#$#$#$#$#$#$#$#$#$#$#$#$#$#$#$#$#$#$#$#$#$#$#$#$#$#$#$#$#$#$#$#$#$#$#$#$#$#$#$#$#$#$#$#$#$#$#$#$#$#$#$#$#$#$#$#$#$#$#$#$#$#$#$#$#$#$#$#$#$#$#$#$#$#$#$#$#$#$#$#$#$#$#$#$#$#$#$#$#$#$#$#$#$#$#$#$#$#$#$#$#$#$#$#$#$#$#$#$#$#$#$#$#$#$#$#$#$#$#$#$#$#$#$#$#$#$#$#$#$#$#$#$#$#$#$#$#$#$#$#$#$#$#$#$#$#$#$#$#$#$#$#$#$#$#$#$#$#$#$#$#$#$#$#$#$#$#$#$#$#$#$#$#$#$#$#$#$#$#$#$#$#$#$#$#$#$#$#$#$#$#$#$#$#$#$#$#$#$#$#$#$#$#$#$#$#$#$#$#$#$#$#$#$#$#$#$#$#$#$#$#$#$#$#$#$#$#$#$#$#$#$#$#$#$#$#$#$#$#$#$#$#$#$#$#$#$#$#$#$#$#$#$#$#$#$#$#$#$#$#$#$#$#$#$#$#$#$#$#$#$#$#$#$#$#$#$#$#$#$#$#$#$#$#$#$#$#$#$#$#$#$#$#$#$#$#$#$#$#$#$#$#$#$#$#$#$#$#$#$#$#$#$#$#$#$#$#$#$#$#$#$#$#$#$#$#$#$#$#$#$#$#$#$#$#$#$#$#$#$#$#$#$#$#$#$#$#$#$#$#$#$#$#$#$#$#$#$#$#$#$#$#$#$#$#$#$#$#$#$#$#$#$#$#$#$#$#$#$#$#$#$#$#$#$#$#$#$#$#$#$#$#$#$#$#$#$#$#$#$#$#$#$#$#$#$#$#$#$#$#$#$#$#$#$#$#$#$#$#$#$#$#$#$#$#$#$#$#$#$#$#$#$#$#$#$#$#$#$#$#$#$#$#$#$#$#$#$#$#$#$#$#$#$#$#$#$#$#$#$#$#$#$#$#$#$#$#$#$#$#$#$#$#$#$#$#$#$#$#$#$#$#$#$#$#$#$#$#$#$#$#$#$#$#$#$#$#$#$#$#$#$#$#$#$#$#$#$#$#$#$#$#$#$#$#$#$#$#$#$#$#$#$#$#$#$#$#$#$#$#$#$#$#$#$#$#$#$#$#$#$#$#$#$#$#$#$#$#$#$#$#$#$#$#$#$#$#$#$#$#$#$#$#$#$#$#$#$#$#$#$#$#$#$#$#$#$#$#$#$#$#$#$#$#$#$#$#$#$#$#$#$#$#$#$#$#$#$#$#$#$#$#$#$#$#$#$#$#$#$#$#$#$#$#$#$#$#$#$#$#$#$#$#$#$#$#$#$#$#$#$#$#$#$#$#$#$#$#$#$#$#$#$#$#$#$#$#$#$#$#$#$#$#$#$#$#$#$#$#$#$#$#$#$#$#$#$#$#$#$#$#$#$#$#$#$#$#$#$#$#$#$#$#$#$#$#$#$#$#$#$#$#$#$#$#$#$#$#$#$#$#$#$#$#$#$#$#$#$#$#$#$#$#$#$#$#$#$#$#$#$#$#$#$#$#$#$#$#$#$#$#$#$#$#$#$#$#$#$#$#$#$#$#$#$#$#$#$#$#$#$#$#$#$#$#$#$#$#$#$#$#$#$#$#$#$#$#$#$#$#\u0015X", "pjlt';\\]`pjlt';\\]`pjlt';\\]`pjlt';\\]`pjlt';\\]`pjlt';\\]`pjlt';\\]`pjlt';\\]`pjlt';\\]`pjlt';\\]`pjlt';\\]`pjlt';\\]`pjlt';\\]`pjlt';\\]`pjlt';\\]`pjlt';\\]`pjlt';\\]`pjlt';\\]`pjlt';\\]`pjlt';\\]`pjlt';\\]`pjlt';\\]`pjlt';\\]`pjlt';\\]`pjlt';\\]`pjlt';\\]`pjlt';\\]`pjlt';\\]`pjlt';\\]`pjlt';\\]`pjlt';\\]`pjlt';\\]`pjlt';\\]`pjlt';\\]`pjlt';\\]`pjlt';\\]`pjlt';\\]`pjlt';\\]`pjlt';\\]`pjlt';\\]`pjlt';\\]`pjlt';\\]`pjlt';\\]`pjlt';\\]`pjlt';\\]`pjlt';\\]`pjlt';\\]`pjlt';\\]`pjlt';\\]`pjlt';\\]`pjlt';\\]`pjlt';\\]`pjlt';\\]`pjlt';\\]`pjlt';\\]`pjlt';\\]`pjlt';\\]`pjlt';\\]`pjlt';\\]`pjlt';\\]`pjlt';\\]`pjlt';\\]`pjlt';\\]`pjlt';\\]`pjlt';\\]`pjlt';\\]`pjlt';\\]`pjlt';\\]`pjlt';\\]`pjlt';\\]`pjlt';\\]`pjlt';\\]`pjlt';\\]`pjlt';\\]`pjlt';\\]`pjlt';\\]`pjlt';\\]`pjlt';\\]`pjlt';\\]`pjlt';\\]`pjlt';\\]`pjlt';\\]`pjlt';\\]`pjlt';\\]`pjlt';\\]`pjlt';\\]`pjlt';\\]`pjlt';\\]`pjlt';\\]`pjlt';\\]`pjlt';\\]`pjlt';\\]`pjlt';\\]`pjlt';\\]`pjlt';\\]`pjlt';\\]`pjlt';\\]`pjlt';\\]`pjlt';\\]`pjlt';\\]`pjlt';\\]`pjlt';\\]`pjlt';\\]`pjlt';\\]`pjlt';\\]`pjlt';\\]`pjlt';\\]`pjlt';\\]`pjlt';\\]`pjlt';\\]`pjlt';\\]`pjlt';\\]`pjlt';\\]`pjlt';\\]`pjlt';\\]`pjlt';\\]`pjlt';\\]`pjlt';\\]`pjlt';\\]`pjlt';\\]`pjlt';\\]`pjlt';\\]`pjlt';\\]`pjlt';\\]`pjlt';\\]`pjlt';\\]`pjlt';\\]`pjlt';\\]`pjlt';\\]`pjlt';\\]`pjlt';\\]`pjlt';\\]`pjlt';\\]`pjlt';\\]`pjlt';\\]`pjlt';\\]`pjlt';\\]`pjlt';\\]`pjlt';\\]`pjlt';\\]`pjlt';\\]`pjlt';\\]`pjlt';\\]`pjlt';\\]`pjlt';\\]`pjlt';\\]`pjlt';\\]`pjlt';\\]`pjlt';\\]`pjlt';\\]`pjlt';\\]`pjlt';\\]`pjlt';\\]`pjlt';\\]`pjlt';\\]`pjlt';\\]`pjlt';\\]`pjlt';\\]`pjlt';\\]`pjlt';\\]`pjlt';\\]`pjlt';\\]`pjlt';\\]`pjlt';\\]`pjlt';\\]`pjlt';\\]`pjlt';\\]`pjlt';\\]`pjlt';\\]`pjlt';\\]`pjlt';\\]`pjlt';\\]`pjlt';\\]`pjlt';\\]`pjlt';\\]`pjlt';\\]`pjlt';\\]`pjlt';\\]`pjlt';\\]`pjlt';\\]`pjlt';\\]`pjlt';\\]`pjlt';\\]`pjlt';\\]`pjlt';\\]`pjlt';\\]`pjlt';\\]`pjlt';\\]`pjlt';\\]`pjlt';\\]`pjlt';\\]`pjlt';\\]`pjlt';\\]`pjlt';\\]`pjlt';\\]`pjlt';\\]`pjlt';\\]`pjlt';\\]`pjlt';\\]`pjlt';\\]`pjlt';\\]`pjlt';\\]`pjlt';\\]`pjlt';\\]`pjlt';\\]`pjlt';\\]`pjlt';\\]`pjlt';\\]`pjlt';\\]`pjlt';\\]`pjlt';\\]`pjlt';\\]`pjlt';\\]`pjlt';\\]`pjlt';\\]`pjlt';\\]`pjlt';\\]`pjlt';\\]`pjlt';\\]`pjlt';\\]`pjlt';\\]`pjlt';\\]`pjlt';\\]`pjlt';\\]`pjlt';\\]`pjlt';\\]`pjlt';\\]`pjlt';\\]`pjlt';\\]`pjlt';\\]`pjlt';\\]`pjlt';\\]`pjlt';\\]`pjlt';\\]`pjlt';\\]`pjlt';\\]`pjlt';\\]`pjlt';\\]`pjlt';\\]`pjlt';\\]`pjlt';\\]`pjlt';\\]`pjlt';\\]`pjlt';\\]`pjlt';\\]`pjlt';\\]`pjlt';\\]`pjlt';\\]`pjlt';\\]`pjlt';\\]`pjlt';\\]`pjlt';\\]`pjlt';\\]`pjlt';\\]`pjlt';\\]`pjlt';\\]`pjlt';\\]`pjlt';\\]`pjlt';\\]`pjlt';\\]`pjlt';\\]`pjlt';\\]`pjlt';\\]`pjlt';\\]`pjlt';\\]`pjlt';\\]`pjlt';\\]`pjlt';\\]`pjlt';\\]`pjlt';\\]`pjlt';\\]`pjlt';\\]`pjlt';\\]`pjlt';\\]`pjlt';\\]`pjlt';\\]`pjlt';\\]`pjlt';\\]`pjlt';\\]`pjlt';\\]`pjlt';\\]`pjlt';\\]`pjlt';\\]`pjlt';\\]`pjlt';\\]`pjlt';\\]`pjlt';\\]`pjlt';\\]`pjlt';\\]`pjlt';\\]`pjlt';\\]`pjlt';\\]`pjlt';\\]`pjlt';\\]`pjlt';\\]`pjlt';\\]`pjlt';\\]`pjlt';\\]`pjlt';\\]`pjlt';\\]`pjlt';\\]`pjlt';\\]`pjlt';\\]`pjlt';\\]`pjlt';\\]`pjlt';\\]`pjlt';\\]`pjlt';\\]`pjlt';\\]`pjlt';\\]`pjlt';\\]`pjlt';\\]`pjlt';\\]`pjlt';\\]`pjlt';\\]`pjlt';\\]`pjlt';\\]`pjlt';\\]`pjlt';\\]`pjlt';\\]`pjlt';\\]`pjlt';\\]`pjlt';\\]`pjlt';\\]`pjlt';\\]`pjlt';\\]`pjlt';\\]`pjlt';\\]`pjlt';\\]`pjlt';\\]`pjlt';\\]`pjlt';\\]`pjlt';\\]`pjlt';\\]`pjlt';\\]`pjlt';\\]`pjlt';\\]`pjlt';\\]`pjlt';\\]`pjlt';\\]`pjlt';\\]`pjlt';\\]`pjlt';\\]`pjlt';\\]`pjlt';\\]`pjlt';\\]`pjlt';\\]`pjlt';\\]`pjlt';\\]`pjlt';\\]`pjlt';\\]`pjlt';\\]`pjlt';\\]`pjlt';\\]`pjlt';\\]`pjlt';\\]`pjlt';\\]`pjlt';\\]`pjlt';\\]`pjlt';\\]`pjlt';\\]`pjlt';\\]`pjlt';\\]`pjlt';\\]`pjlt';\\]`pjlt';\\]`pjlt';\\]`pjlt';\\]`pjlt';\\]`pjlt';\\]`pjlt';\\]`pjlt';\\]`pjlt';\\]`pjlt';\\]`pjlt';\\]`pjlt';\\]`pjlt';\\]`pjlt';\\]`pjlt';\\]`pjlt';\\]`pjlt';\\]`pjlt';\\]`pjlt';\\]`pjlt';\\]`pjlt';\\]`pjlt';\\]`pjlt';\\]`pjlt';\\]`pjlt';\\]`pjlt';\\]`pjlt';\\]`pjlt';\\]`pjlt';\\]`pjlt';\\]`pjlt';\\]`pjlt';\\]`pjlt';\\]`pjlt';\\]`pjlt';\\]`pjlt';\\]`pjlt';\\]`pjlt';\\]`pjlt';\\]`pjlt';\\]`pjlt';\\]`pjlt';\\]`pjlt';\\]`pjlt';\\]`pjlt';\\]`pjlt';\\]`pjlt';\\]`pjlt';\\]`pjlt';\\]`pjlt';\\]`pjlt';\\]`pjlt';\\]`pjlt';\\]`pjlt';\\]`pjlt';\\]`pjlt';\\]`pjlt';\\]`pjlt';\\]`pjlt';\\]`pjlt';\\]`pjlt';\\]`pjlt';\\]`pjlt';\\]`pjlt';\\]`pjlt';\\]`pjlt';\\]`pjlt';\\]`pjlt';\\]`pjlt';\\]`pjlt';\\]`pjlt';\\]`pjlt';\\]`pjlt';\\]`pjlt';\\]`pjlt';\\]`pjlt';\\]`pjlt';\\]`pjlt';\\]`pjlt';\\]`pjlt';\\]`pjlt';\\]`pjlt';\\]`pjlt';\\]`pjlt';\\]`pjlt';\\]`pjlt';\\]`pjlt';\\]`pjlt';\\]`pjlt';\\]`pjlt';\\]`pjlt';\\]`pjlt';\\]`pjlt';\\]`pjlt';\\]`pjlt';\\]`pjlt';\\]`pjlt';\\]`pjlt';\\]`pjlt';\\]`pjlt';\\]`pjlt';\\]`pjlt';\\]`pjlt';\\]`pjlt';\\]`pjlt';\\]`pjlt';\\]`pjlt';\\]`pjlt';\\]`pjlt';\\]`pjlt';\\]`pjlt';\\]`pjlt';\\]`pjlt';\\]`pjlt';\\]`pjlt';\\]`pjlt';\\]`pjlt';\\]`pjlt';\\]`pjlt';\\]`pjlt';\\]`pjlt';\\]`pjlt';\\]`pjlt';\\]`pjlt';\\]`pjlt';\\]`pjlt';\\]`pjlt';\\]`pjlt';\\]`pjlt';\\]`pjlt';\\]`pjlt';\\]`pjlt';\\]`pjlt';\\]`pjlt';\\]`pjlt';\\]`pjlt';\\]`pjlt';\\]`pjlt';\\]`pjlt';\\]`pjlt';\\]`pjlt';\\]`pjlt';\\]`pjlt';\\]`pjlt';\\]`pjlt';\\]`pjlt';\\]`pjlt';\\]`pjlt';\\]`pjlt';\\]`pjlt';\\]`pjlt';\\]`pjlt';\\]`pjlt';\\]`pjlt';\\]`pjlt';\\]`pjlt';\\]`pjlt';\\]`pjlt';\\]`pjlt';\\]`pjlt';\\]`pjlt';\\]`pjlt';\\]`pjlt';\\]`pjlt';\\]`pjlt';\\]`pjlt';\\]`pjlt';\\]`pjlt';\\]`pjlt';\\]`pjlt';\\]`pjlt';\\]`pjlt';\\]`pjlt';\\]`pjlt';\\]`pjlt';\\]`pjlt';\\]`pjlt';\\]`pjlt';\\]`pjlt';\\]`pjlt';\\]`pjlt';\\]`pjlt';\\]`pjlt';\\]`pjlt';\\]`pjlt';\\]`pjlt';\\]`pjlt';\\]`pjlt';\\]`pjlt';\\]`pjlt';\\]`pjlt';\\]`pjlt';\\]`pjlt';\\]`pjlt';\\]`pjlt';\\]`pjlt';\\]`pjlt';\\]`pjlt';\\]`pjlt';\\]`pjlt';\\]`pjlt';\\]`pjlt';\\]`pjlt';\\]`pjlt';\\]`pjlt';\\]`pjlt';\\]`pjlt';\\]`pjlt';\\]`pjlt';\\]`pjlt';\\]`pjlt';\\]`pjlt';\\]`pjlt';\\]`pjlt';\\]`pjlt';\\]`pjlt';\\]`pjlt';\\]`pjlt';\\]`pjlt';\\]`pjlt';\\]`pjlt';\\]`pjlt';\\]`pjlt';\\]`pjlt';\\]`pjlt';\\]`pjlt';\\]`pjlt';\\]`pjlt';\\]`pjlt';\\]`pjlt';\\]`pjlt';\\]`pjlt';\\]`pjlt';\\]`pjlt';\\]`pjlt';\\]`pjlt';\\]`pjlt';\\]`pjlt';\\]`pjlt';\\]`pjlt';\\]`pjlt';\\]`pjlt';\\]`pjlt';\\]`pjlt';\\]`pjlt';\\]`pjlt';\\]`pjlt';\\]`pjlt';\\]`pjlt';\\]`pjlt';\\]`pjlt';\\]`pjlt';\\]`pjlt';\\]`pjlt';\\]`pjlt';\\]`pjlt';\\]`pjlt';\\]`pjlt';\\]`pjlt';\\]`pjlt';\\]`pjlt';\\]`pjlt';\\]`pjlt';\\]`pjlt';\\]`pjlt';\\]`pjlt';\\]`pjlt';\\]`pjlt';\\]`pjlt';\\]`pjlt';\\]`pjlt';\\]`pjlt';\\]`pjlt';\\]`pjlt';\\]`pjlt';\\]`pjlt';\\]`pjlt';\\]`pjlt';\\]`pjlt';\\]`pjlt';\\]`pjlt';\\]`pjlt';\\]`pjlt';\\]`pjlt';\\]`pjlt';\\]`pjlt';\\]`pjlt';\\]`pjlt';\\]`pjlt';\\]`pjlt';\\]`pjlt';\\]`pjlt';\\]`pjlt';\\]`pjlt';\\]`pjlt';\\]`pjlt';\\]`pjlt';\\]`pjlt';\\]`pjlt';\\]`pjlt';\\]`pjlt';\\]`pjlt';\\]`pjlt';\\]`pjlt';\\]`pjlt';\\]`pjlt';\\]`pjlt';\\]`pjlt';\\]`pjlt';\\]`pjlt';\\]`pjlt';\\]`pjlt';\\]`pjlt';\\]`pjlt';\\]`pjlt';\\]`pjlt';\\]`pjlt';\\]`pjlt';\\]`pjlt';\\]`pjlt';\\]`pjlt';\\]`pjlt';\\]`pjlt';\\]`pjlt';\\]`pjlt';\\]`pjlt';\\]`pjlt';\\]`pjlt';\\]`pjlt';\\]`pjlt';\\]`pjlt';\\]`pjlt';\\]`pjlt';\\]`pjlt';\\]`pjlt';\\]`pjlt';\\]`pjlt';\\]`pjlt';\\]`pjlt';\\]`pjlt';\\]`pjlt';\\]`pjlt';\\]`pjlt';\\]`pjlt';\\]`pjlt';\\]`pjlt';\\]`pjlt';\\]`pjlt';\\]`pjlt';\\]`pjlt';\\]`pjlt';\\]`pjlt';\\]`pjlt';\\]`pjlt';\\]`pjlt';\\]`pjlt';\\]`pjlt';\\]`pjlt';\\]`pjlt';\\]`pjlt';\\]`pjlt';\\]`pjlt';\\]`pjlt';\\]`pjlt';\\]`pjlt';\\]`pjlt';\\]`pjlt';\\]`pjlt';\\]`pjlt';\\]`pjlt';\\]`pjlt';\\]`pjlt';\\]`pjlt';\\]`pjlt';\\]`pjlt';\\]`pjlt';\\]`pjlt';\\]`pjlt';\\]`pjlt';\\]`pjlt';\\]`pjlt';\\]`pjlt';\\]`pjlt';\\]`pjlt';\\]`pjlt';\\]`pjlt';\\]`pjlt';\\]`pjlt';\\]`pjlt';\\]`pjlt';\\]`pjlt';\\]`pjlt';\\]`pjlt';\\]`pjlt';\\]`pjlt';\\]`pjlt';\\]`pjlt';\\]`pjlt';\\]`pjlt';\\]`pjlt';\\]`pjlt';\\]`pjlt';\\]`pjlt';\\]`pjlt';\\]`pjlt';\\]`pjlt';\\]`pjlt';\\]`pjlt';\\]`pjlt';\\]`pjlt';\\]`pjlt';\\]`pjlt';\\]`pjlt';\\]`pjlt';\\]`pjlt';\\]`pjlt';\\]`pjlt';\\]`pjlt';\\]`pjlt';\\]`pjlt';\\]`pjlt';\\]`pjlt';\\]`pjlt';\\]`pjlt';\\]`pjlt';\\]`pjlt';\\]`pjlt';\\]`pjlt';\\]`pjlt';\\]`pjlt';\\]`pjlt';\\]`pjlt';\\]`pjlt';\\]`pjlt';\\]`pjlt';\\]`pjlt';\\]`pjlt';\\]`pjlt';\\]`pjlt';\\]`pjlt';\\]`pjlt';\\]`pjlt';\\]`pjlt';\\]`pjlt';\\]`pjlt';\\]`pjlt';\\]`pjlt';\\]`pjlt';\\]`pjlt';\\]`pjlt';\\]`pjlt';\\]`pjlt';\\]`pjlt';\\]`pjlt';\\]`pjlt';\\]`pjlt';\\]`pjlt';\\]`pjlt';\\]`pjlt';\\]`pjlt';\\]`pjlt';\\]`pjlt';\\]`pjlt';\\]`pjlt';\\]`pjlt';\\]`pjlt';\\]`pjlt';\\]`pjlt';\\]`pjlt';\\]`pjlt';\\]`pjlt';\\]`pjlt';\\]`pjlt';\\]`pjlt';\\]`pjlt';\\]`pjlt';\\]`pjlt';\\]`pjlt';\\]`pjlt';\\]`pjlt';\\]`pjlt';\\]`pjlt';\\]`pjlt';\\]`pjlt';\\]`pjlt';\\]`pjlt';\\]`pjlt';\\]`pjlt';\\]`pjlt';\\]`pjlt';\\]`pjlt';\\]`pjlt';\\]`pjlt';\\]`pjlt';\\]`pjlt';\\]`pjlt';\\]`pjlt';\\]`pjlt';\\]`pjlt';\\]`pjlt';\\]`pjlt';\\]`pjlt';\\]`pjlt';\\]`pjlt';\\]`pjlt';\\]`pjlt';\\]`pjlt';\\]`pjlt';\\]`pjlt';\\]`pjlt';\\]`pjlt';\\]`pjlt';\\]`pjlt';\\]`pjlt';\\]`pjlt';\\]`pjlt';\\]`pjlt';\\]`pjlt';\\]`pjlt';\\]`pjlt';\\]`pjlt';\\]`pjlt';\\]`pjlt';\\]`pjlt';\\]`pjlt';\\]`pjlt';\\]`pjlt';\\]`pjlt';\\]`pjlt';\\]`pjlt';\\]`pjlt';\\]`pjlt';\\]`pjlt';\\]`pjlt';\\]`pjlt';\\]`pjlt';\\]`pjlt';\\]`pjlt';\\]`pjlt';\\]`pjlt';\\]`pjlt';\\]`pjlt';\\]`pjlt';\\]`pjlt';\\]`pjlt';\\]`pjlt';\\]`pjlt';\\]`pjlt';\\]`pjlt';\\]`pjlt';\\]`pjlt';\\]`pjlt';\\]`pjlt';\\]`pjlt';\\]`pjlt';\\]`pjlt';\\]`pjlt';\\]`pjlt';\\]`pjlt';\\]`pjlt';\\]`pjlt';\\]`pjlt';\\]`pjlt';\\]`pjlt';\\]`pjlt';\\]`pjlt';\\]`pjlt';\\]`pjlt';\\]`pjlt';\\]`pjlt';\\]`pjlt';\\]`pjlt';\\]`pjlt';\\]`pjlt';\\]`pjlt';\\]`pjlt';\\]`pjlt';\\]`pjlt';\\]`pjlt';\\]`pjlt';\\]`pjlt';\\]`pjlt';\\]`pjlt';\\]`pjlt';\\]`pjlt';\\]`pjlt';\\]`pjlt';\\]`pjlt';\\]`pjlt';\\]`pjlt';\\]`pjlt';\\]`pjlt';\\]`pjlt';\\]`pjlt';\\]`pjlt';\\]`pjlt';\\]`pjlt';\\]`pjlt';\\]`pjlt';\\]`pjlt';\\]`pjlt';\\]`pjlt';\\]`pjlt';\\]`pjlt';\\]`pjlt';\\]`pjlt';\\]`pjlt';\\]`pjlt';\\]`pjlt';\\]`pjlt';\\]`pjlt';\\]`pjlt';\\]`pjlt';\\]`pjlt';\\]`pjlt';\\]`pjlt';\\]`pjlt';\\]`pjlt';\\]`pjlt';\\]`pjlt';\\]`pjlt';\\]`pjlt';\\]`pjlt';\\]`pjlt';\\]`pjlt';\\]`pjlt';\\]`pjlt';\\]`pjlt';\\]`pjlt';\\]`pjlt';\\]`pjlt';\\]`pjlt';\\]`pjlt';\\]`pjlt';\\]`pjlt';\\]`pjlt';\\]`‡\b", "~~~~~~~~~~~~~~~~~~~~~~~~~~~~~~~~~~~~~~~~~~~~~~~~~~~~~~~~~~~~~~~~~~~~~~~~~~~~~~~~~~~~~~~~~~~~~~~~~~~~~~~~~~~~~~~~~~~~~~~~~~~~~~~~~~~~~~~~~~~~~~~~~~~~~~~~~~~~~~~~~~~~~~~~~~~~~~~~~~~~~~~~~~~~~~~~~~~~~~~~~~~~~~~~~~~~~~~~~~~~~~~~~~~~~~~~~~~~~~~~~~~~~~~~~~~~~~~~~~~~~~~~~~~~~~~~~~~~~~~~~~~~~~~~~~~~~~~~~~~~~~~~~~~~~~~~~~~~~~~~~~~~~~~~~~~~~~~~~~~~~~~~~~~~~~~~~~~~~~~~~~~~~~~~~~~~~~~~~~~~~~~~~~~~~~~~~~~~~~~~~~~~~~~~~~~~~~~~~~~~~~~~~~~~~~~~~~~~~~~~~~~~~~~~~~~~~~~~~~~~~~~~~~~~~~~~~~~~~~~~~~~~~~~~~~~~~~~~~~~~~~~~~~~~~~~~~~~~~~~~~~~~~~~~~~~~~~~~~~~~~~~~~~~~~~~~~~~~~~~~~~~~~~~~~~~~~~~~~~~~~~~~~~~~~~~~~~~~~~~~~~~~~~~~~~~~~~~~~~~~~~~~~~~~~~~~~~~~~~~~~~~~~~~~~~~~~~~~~~~~~~~~~~~~~~~~~~~~~~~~~~~~~~~~~~~~~~~~~~~~~~~~~~~~~~~~~~~~~~~~~~~~~~~~~~~~~~~~~~~~~~~~~~~~~~~~~~~~~~~~~~~~~~~~~~~~~~~~~~~~~~~~~~~~~~~~~~~~~~~~~~~~~~~~~~~~~~~~~~~~~~~~~~~~~~~~~~~~~~~~~~~~~~~~~~~~~~~~~~~~~~~~~~~~~~~~~~~~~~~~~~~~~~~~~~~~~~~~~~~~~~~~~~~~~~~~~~~~~~~~~~~~~~~~~~~~~~~~~~~~~~~~~~~~~~~~~~~~~~~~~~~~~~~~~~~~~~~~~~~~~~~~~~~~~~~~~~~~~~~~ì0", "LabVIEWLabVIEWLabVIEWLabVIEWLabVIEWLabVIEWLabVIEWLabVIEWLabVIEWLabVIEWLabVIEWLabVIEWLabVIEWLabVIEWLabVIEWLabVIEWLabVIEWLabVIEWLabVIEWLabVIEWLabVIEWLabVIEWLabVIEWLabVIEWLabVIEWLabVIEWLabVIEWLabVIEWLabVIEWLabVIEWLabVIEWLabVIEWLabVIEWLabVIEWLabVIEWLabVIEWLabVIEWLabVIEWLabVIEWLabVIEWLabVIEWLabVIEWLabVIEWLabVIEWLabVIEWLabVIEWLabVIEWLabVIEWLabVIEWLabVIEWLabVIEWLabVIEWLabVIEWLabVIEWLabVIEWLabVIEWLabVIEWLabVIEWLabVIEWLabVIEWLabVIEWLabVIEWLabVIEWLabVIEWLabVIEWLabVIEWLabVIEWLabVIEWLabVIEWLabVIEWLabVIEWLabVIEWLabVIEWLabVIEWLabVIEWLabVIEWLabVIEWLabVIEWLabVIEWLabVIEWLabVIEWLabVIEWLabVIEWLabVIEWLabVIEWLabVIEWLabVIEWLabVIEWLabVIEWLabVIEWLabVIEWLabVIEWLabVIEWLabVIEWLabVIEWLabVIEWLabVIEWLabVIEWLabVIEWLabVIEWLabVIEWLabVIEWLabVIEWLabVIEWLabVIEWLabVIEWLabVIEWLabVIEWLabVIEWLabVIEWLabVIEWLabVIEWLabVIEWLabVIEWLabVIEWLabVIEWLabVIEWLabVIEWLabVIEWLabVIEWLabVIEWLabVIEWLabVIEWLabVIEWLabVIEWLabVIEWLabVIEWLabVIEWLabVIEWLabVIEWLabVIEWLabVIEWLabVIEWLabVIEWLabVIEWLabVIEWLabVIEWLabVIEWLabVIEWLabVIEWLabVIEWLabVIEWLabVIEWLabVIEWLabVIEWLabVIEWLabVIEWLabVIEWLabVIEWLabVIEWLabVIEWLabVIEWLabVIEWLabVIEWLabVIEWLabVIEWLabVIEWLabVIEWLabVIEWLabVIEWLabVIEWLabVIEWLabVIEWLabVIEWLabVIEWLabVIEWLabVIEWLabVIEWLabVIEWLabVIEWLabVIEWLabVIEWLabVIEWLabVIEWLabVIEWLabVIEWLabVIEWLabVIEWLabVIEWLabVIEWLabVIEWLabVIEWLabVIEWLabVIEWLabVIEWLabVIEWLabVIEWLabVIEWLabVIEWLabVIEWLabVIEWLabVIEWLabVIEWLabVIEWLabVIEWLabVIEWLabVIEWLabVIEWLabVIEWLabVIEWLabVIEWLabVIEWLabVIEWLabVIEWLabVIEWLabVIEWLabVIEWLabVIEWLabVIEWLabVIEWLabVIEWLabVIEWLabVIEWLabVIEWLabVIEWLabVIEWLabVIEWLabVIEWLabVIEWLabVIEWLabVIEWLabVIEWLabVIEWLabVIEWLabVIEWLabVIEWLabVIEWLabVIEWLabVIEWLabVIEWLabVIEWLabVIEWLabVIEWLabVIEWLabVIEWLabVIEWLabVIEWLabVIEWLabVIEWLabVIEWLabVIEWLabVIEWLabVIEWLabVIEWLabVIEWLabVIEWLabVIEWLabVIEWLabVIEWLabVIEWLabVIEWLabVIEWLabVIEWLabVIEWLabVIEWLabVIEWLabVIEWLabVIEWLabVIEWLabVIEWLabVIEWLabVIEWLabVIEWLabVIEWLabVIEWLabVIEWLabVIEWLabVIEWLabVIEWLabVIEWLabVIEWLabVIEWLabVIEWLabVIEWLabVIEWLabVIEWLabVIEWLabVIEWLabVIEWLabVIEWLabVIEWLabVIEWLabVIEWLabVIEWLabVIEWLabVIEWLabVIEWLabVIEWLabVIEWLabVIEWLabVIEWLabVIEWLabVIEWLabVIEWLabVIEWLabVIEWLabVIEWLabVIEWLabVIEWLabVIEWLabVIEWLabVIEWLabVIEWLabVIEWLabVIEWLabVIEWLabVIEWLabVIEWLabVIEWLabVIEWLabVIEWLabVIEWLabVIEWLabVIEWLabVIEWLabVIEWLabVIEWLabVIEWLabVIEWLabVIEWLabVIEWLabVIEWLabVIEWLabVIEWLabVIEWLabVIEWLabVIEWLabVIEWLabVIEWLabVIEWLabVIEWLabVIEWLabVIEWLabVIEWLabVIEWLabVIEWLabVIEWLabVIEWLabVIEWLabVIEWLabVIEWLabVIEWLabVIEWLabVIEWLabVIEWLabVIEWLabVIEWLabVIEWLabVIEWLabVIEWLabVIEWLabVIEWLabVIEWLabVIEWLabVIEWLabVIEWLabVIEWLabVIEWLabVIEWLabVIEWLabVIEWLabVIEWLabVIEWLabVIEWLabVIEWLabVIEWLabVIEWLabVIEWLabVIEWLabVIEWLabVIEWLabVIEWLabVIEWLabVIEWLabVIEWLabVIEWLabVIEWLabVIEWLabVIEWLabVIEWLabVIEWLabVIEWLabVIEWLabVIEWLabVIEWLabVIEWLabVIEWLabVIEWLabVIEWLabVIEWLabVIEWLabVIEWLabVIEWLabVIEWLabVIEWLabVIEWLabVIEWLabVIEWLabVIEWLabVIEWLabVIEWLabVIEWLabVIEWLabVIEWLabVIEWLabVIEWLabVIEWLabVIEWLabVIEWLabVIEWLabVIEWLabVIEWLabVIEWLabVIEWLabVIEWLabVIEWLabVIEWLabVIEWLabVIEWLabVIEWLabVIEWLabVIEWLabVIEWLabVIEWLabVIEWLabVIEWLabVIEWLabVIEWLabVIEWLabVIEWLabVIEWLabVIEWLabVIEWLabVIEWLabVIEWLabVIEWLabVIEWLabVIEWLabVIEWLabVIEWLabVIEWLabVIEWLabVIEWLabVIEWLabVIEWLabVIEWLabVIEWLabVIEWLabVIEWLabVIEWLabVIEWLabVIEWLabVIEWLabVIEWLabVIEWLabVIEWLabVIEWLabVIEWLabVIEWLabVIEWLabVIEWLabVIEWLabVIEWLabVIEWLabVIEWLabVIEWLabVIEWLabVIEWLabVIEWLabVIEWLabVIEWLabVIEWLabVIEWLabVIEWLabVIEWLabVIEWLabVIEWLabVIEWLabVIEWLabVIEWLabVIEWLabVIEWLabVIEWLabVIEWLabVIEWLabVIEWLabVIEWLabVIEWLabVIEWLabVIEWLabVIEWLabVIEWLabVIEWLabVIEWLabVIEWLabVIEWLabVIEWLabVIEWLabVIEWLabVIEWLabVIEWLabVIEWLabVIEWLabVIEWLabVIEWLabVIEWLabVIEWLabVIEWLabVIEWLabVIEWLabVIEWLabVIEWLabVIEWLabVIEWLabVIEWLabVIEWLabVIEWLabVIEWLabVIEWLabVIEWLabVIEWLabVIEWLabVIEWLabVIEWLabVIEWLabVIEWLabVIEWLabVIEWLabVIEWLabVIEWLabVIEWLabVIEWLabVIEWLabVIEWLabVIEWLabVIEWLabVIEWLabVIEWLabVIEWLabVIEWLabVIEWLabVIEWLabVIEWLabVIEWLabVIEWLabVIEWLabVIEWLabVIEWLabVIEWLabVIEWLabVIEWLabVIEWLabVIEWLabVIEWLabVIEWLabVIEWLabVIEWLabVIEWLabVIEWLabVIEWLabVIEWLabVIEWLabVIEWLabVIEWLabVIEWLabVIEWLabVIEWLabVIEWLabVIEWLabVIEWLabVIEWLabVIEWLabVIEWLabVIEWLabVIEWLabVIEWLabVIEWLabVIEWLabVIEWLabVIEWLabVIEWLabVIEWLabVIEWLabVIEWLabVIEWLabVIEWLabVIEWLabVIEWLabVIEWLabVIEWLabVIEWLabVIEWLabVIEWLabVIEWLabVIEWLabVIEWLabVIEWLabVIEWLabVIEWLabVIEWLabVIEWLabVIEWLabVIEWLabVIEWLabVIEWLabVIEWLabVIEWLabVIEWLabVIEWLabVIEWLabVIEWLabVIEWLabVIEWLabVIEWLabVIEWLabVIEWLabVIEWLabVIEWLabVIEWLabVIEWLabVIEWLabVIEWLabVIEWLabVIEWLabVIEWLabVIEWLabVIEWLabVIEWLabVIEWLabVIEWLabVIEWLabVIEWLabVIEWLabVIEWLabVIEWLabVIEWLabVIEWLabVIEWLabVIEWLabVIEWLabVIEWLabVIEWLabVIEWLabVIEWLabVIEWLabVIEWLabVIEWLabVIEWLabVIEWLabVIEWLabVIEWLabVIEWLabVIEWLabVIEWLabVIEWLabVIEWLabVIEWLabVIEWLabVIEWLabVIEWLabVIEWLabVIEWLabVIEWLabVIEWLabVIEWLabVIEWLabVIEWLabVIEWLabVIEWLabVIEWLabVIEWLabVIEWLabVIEWLabVIEWLabVIEWLabVIEWLabVIEWLabVIEWLabVIEWLabVIEWLabVIEWLabVIEWLabVIEWLabVIEWLabVIEWLabVIEWLabVIEWLabVIEWLabVIEWLabVIEWLabVIEWLabVIEWLabVIEWLabVIEWLabVIEWLabVIEWLabVIEWLabVIEWLabVIEWLabVIEWLabVIEWLabVIEWLabVIEWLabVIEWLabVIEWLabVIEWLabVIEWLabVIEWLabVIEWLabVIEWLabVIEWLabVIEWLabVIEWLabVIEWLabVIEWLabVIEWLabVIEWLabVIEWLabVIEWLabVIEWLabVIEWLabVIEWLabVIEWLabVIEWLabVIEWLabVIEWLabVIEWLabVIEWLabVIEWLabVIEWLabVIEWLabVIEWLabVIEWLabVIEWLabVIEWLabVIEWLabVIEWLabVIEWLabVIEWLabVIEWLabVIEWLabVIEWLabVIEWLabVIEWLabVIEWLabVIEWLabVIEWLabVIEWLabVIEWLabVIEWLabVIEWLabVIEWLabVIEWLabVIEWLabVIEWLabVIEWLabVIEWLabVIEWLabVIEWLabVIEWLabVIEWLabVIEWLabVIEWLabVIEWLabVIEWLabVIEWLabVIEWLabVIEWLabVIEWLabVIEWLabVIEWLabVIEWLabVIEWLabVIEWLabVIEWLabVIEWLabVIEWLabVIEWLabVIEWLabVIEWLabVIEWLabVIEWLabVIEWLabVIEWLabVIEWLabVIEWLabVIEWLabVIEWLabVIEWLabVIEWLabVIEWLabVIEWLabVIEWLabVIEWLabVIEWLabVIEWLabVIEWLabVIEWLabVIEWLabVIEWLabVIEWLabVIEWLabVIEWLabVIEWLabVIEWLabVIEWLabVIEWLabVIEWLabVIEWLabVIEWLabVIEWLabVIEWLabVIEWLabVIEWLabVIEWLabVIEWLabVIEWLabVIEWLabVIEWLabVIEWLabVIEWLabVIEWLabVIEWLabVIEWLabVIEWLabVIEWLabVIEWLabVIEWLabVIEWLabVIEWLabVIEWLabVIEWLabVIEWLabVIEWLabVIEWLabVIEWLabVIEWLabVIEWLabVIEWLabVIEWLabVIEWLabVIEWLabVIEWLabVIEWLabVIEWLabVIEWLabVIEWLabVIEWLabVIEWLabVIEWLabVIEWLabVIEWLabVIEWLabVIEWLabVIEWLabVIEWLabVIEWLabVIEWLabVIEWLabVIEWLabVIEWLabVIEWLabVIEWLabVIEWLabVIEWLabVIEWLabVIEWLabVIEWLabVIEWLabVIEWLabVIEWLabVIEWLabVIEWLabVIEWLabVIEWLabVIEWLabVIEWLabVIEWLabVIEWLabVIEWLabVIEWLabVIEWLabVIEWLabVIEWLabVIEWLabVIEWLabVIEWLabVIEWLabVIEWLabVIEWLabVIEWLabVIEWLabVIEWLabVIEWLabVIEWLabVIEWLabVIEWLabVIEWLabVIEWLabVIEWLabVIEWLabVIEWLabVIEWLabVIEWLabVIEWLabVIEWLabVIEWLabVIEWLabVIEWLabVIEWLabVIEWLabVIEWLabVIEWLabVIEWLabVIEWLabVIEWLabVIEWLabVIEWLabVIEWLabVIEWLabVIEWLabVIEWLabVIEWLabVIEWLabVIEWLabVIEWLabVIEWLabVIEWLabVIEWLabVIEWLabVIEWLabVIEWLabVIEWLabVIEWLabVIEWLabVIEWLabVIEWLabVIEWLabVIEWLabVIEWLabVIEWLabVIEWLabVIEWLabVIEWLabVIEWLabVIEWLabVIEWLabVIEWLabVIEWLabVIEWLabVIEWLabVIEWLabVIEWLabVIEWLabVIEWLabVIEWLabVIEWLabVIEWLabVIEWLabVIEWLabVIEWLabVIEWLabVIEWLabVIEWLabVIEWLabVIEWLabVIEWLabVIEWLabVIEWLabVIEWLabVIEWLabVIEWLabVIEWLabVIEWLabVIEWLabVIEWLabVIEWLabVIEWLabVIEWLabVIEWLabVIEWLabVIEWLabVIEWLabVIEWLabVIEWLabVIEWLabVIEWLabVIEWLabVIEWLabVIEWLabVIEWLabVIEWLabVIEWLabVIEWLabVIEWLabVIEWLabVIEWLabVIEWLabVIEWLabVIEWñ\u0010"]]  # Expected Array
      w7 = string[] ["QWERTYDSA", "~~w", "abcd", "__dsa/.432", "$#", "pjlt';\\]`", "~", "LabVIEW"]  # String IN Array
      w8 = bool[] [TRUE, FALSE]  # PAD Array
      n2 = for {
        tunnel: [w21] -> w10 mode=indexing
        shift-right: [w20] -> w9
        shift-left: w11 -> [w22]
        tunnel: w8 -> [w19] mode=indexing
        tunnel: w7 -> [w18]
        tunnel: w6 -> [w17]
        tunnel: [w16] -> w5 mode=indexing
        i -> [w15]
        n3 = for {
          tunnel: w18 -> [w30] mode=indexing
          tunnel: w22 -> [w29]
          tunnel: [w26] -> w20
          tunnel: [w25] -> w21 mode=indexing
          tunnel: w19 -> [w28]
          # "The loop has 1000 iterations to ensure that the passed data\ndoes not fit in U16 representation"
          n4 = for {
            N: 1000 -> [_]
            shift-right: [w35] -> w27
            shift-left: "" -> [w34]
            tunnel: w30 -> [w33]
            n5 = Concatenate Strings(w33, w34) -> (w35:string)
          }
          n6 = call-dynamic "Add Protection.vi"("error in (no error)"=w29, "Pad"=w28, "String in"=w27, "Checksum U16 in"="Checksum U16 in") -> ("error out"=w26:errorcluster, "String out"=w25:string, "Checksum U16 out"=→"Checksum U16 out":refnum<class "Checksum U16.lvclass">)  [unwired: 5 in]
        }
        n7 = Index Array "Index Array"(array=w17, index (row)=w15) -> (element=w16:string[])  [unwired: 1 in]
      }
      n8 = call-dynamic "passIfEqual.vi"("error in (no error)"=w9, "y"=w10, "x"=w5, "TestCase in"=w12) -> ("error out"=w14:errorcluster, "TestCase out"=w13:refnum<class "Protections Unit Tests.lvclass">)  [unwired: 6 in]
    }
    frame Disabled {
      # "skip test result while test is under development"
      n9 = call <vilib>:"skip.vi"("error in (no error)"=w36, "TestCase in"=w39) -> ("error out"=w38:errorcluster, "TestCase out"=w37:refnum<class "Protections Unit Tests.lvclass">)  [unwired: 8 in]
    }
  }
  "error out" <- w3
  "TestCase out" <- w1
